vi "Q14070-B030主界面   曲线分布保存.vi"() -> ()   [LabVIEW 2013]
uses:
  <vilib>/printing/EasyPrintingControls.llb/contents.ctl
  <vilib>/printing/EasyPrintingControls.llb/report_type.ctl
  <vilib>/Utility/NIReport.llb/NI_report.lvclass
  <vilib>/printing/EasyPrinting.llb/Easy Print VI Panel or Documentation (path).vi
  <vilib>/Utility/file.llb/Write To Spreadsheet File (DBL).vi
  PCI8622_32.dll
  <vilib>/Utility/NIReport.llb/NI_ReportGenerationCore.lvlib
panel:
  in  "返工次数":dbl
  in  "结束时间":string
  in  "开始时间":string
  out "本工位合格":bool
  out "本工位完成":bool
  out "压衬套伺服压装速度":dbl
  out "压衬套伺服快进速度":dbl
  out "压垫片伺服压装速度":dbl
  out "压垫片伺服快进速度":dbl
  out "压轴承伺服压装速度":dbl
  out "压轴承伺服快进速度":dbl
  in  "本工位放行 7":bool
  in  "本工位放行 6":bool
  in  "本工位放行 5":bool
  in  "本工位放行 4":bool
  in  "压轴承快进位至压装位":bool
  in  "压轴承原位至快进位":bool
  out "压衬套手动走位设置":dbl
  out "压垫片手动走位设置":dbl
  out "压轴承手动走位设置":dbl
  in  "轴承上料工步":u32 caption="工步号1"
  out "轴承上料工步提示":string
  out "压衬套伺服压装位置":dbl
  out "压衬套伺服快进位置":dbl
  out "压垫片伺服压装位置":dbl
  out "压垫片伺服快进位置":dbl
  out "压轴承伺服压装位置":dbl
  out "压轴承伺服快进位置":dbl
  out "压轴承伺服压头位置":dbl
  out "error out":errorcluster
  out "压衬套参数保存错误":errorcluster
  out "压垫片参数保存错误":errorcluster
  in  "压轴承停止完成":bool
  in  "压垫片停止完成":bool
  in  "压衬套停止完成":bool
  in  "预压紧气缸复位":bool
  in  "夹爪全体气缸复位":bool
  in  "电动缸全复位":bool
  in  "电动缸全回零":bool
  in  "工位单循环":bool
  out "压衬套压力数组":dbl[](array[numeric])
  out "压衬套位移数组":dbl[](array[numeric])
  out "压垫片压力数组":dbl[](array[numeric])
  out "压垫片位移数组":dbl[](array[numeric])
  out "压轴承位移数组":dbl[](array[numeric])
  out "压轴承压力数组":dbl[](array[numeric])
  out "压衬套位移":dbl format="%#.3g"
  out "压衬套压力":dbl format="%#.3g"
  out "压垫片位移":dbl format="%#.3g"
  out "压垫片压力":dbl format="%#.3g"
  out "压轴承位移":dbl format="%#.3g"
  out "压轴承压力":dbl format="%#.3g"
  in  "产品ID字符串位数":dbl
  out "报警工步号":u32 caption="工步号1"
  out "报警提示":string
  in  "产品ID":string="201209190001"
  in  "员工ID":string
  out "员工姓名":string
  out "压轴承参数保存错误":errorcluster
  out "传感器保存错误":errorcluster
  in  "报警清除":bool
  in  "参数加载":bool
  in  "型号选择":u32(ring) items=["J706", "J709"]
  out "参数加载错误":errorcluster
  in  "停止":bool
  out "ADODB._Connection Out":refnum<k7>
  out "参数查询错误":errorcluster
  in  "联线按钮":bool
  out "通讯状态":bool
  in  "选项卡控件":T1(tab)
  out "压轴承换向压力(KN)":dbl format="%#.1f"
  out "压轴承压力报警":bool
  out "压轴承监控点压力2(mm)":dbl format="%#.2f"
  out "压轴承监控点压力1(mm)":dbl format="%#.2f"
  out "压轴承区域最大位移1(mm)":dbl format="%#.1f"
  out "压轴承区域最小位移1(mm)":dbl format="%#.1f"
  out "压轴承区域最大压力1(KN)":dbl format="%#.3f"
  out "压轴承区域最小压力1(KN)":dbl format="%#.3f"
  out "压轴承区域最大位移2(mm)":dbl format="%#.1f"
  out "压轴承区域最小位移2(mm)":dbl format="%#.1f"
  out "压轴承区域最大压力2(KN)":dbl format="%#.3f"
  out "压轴承区域最小压力2(KN)":dbl format="%#.3f"
  out "压轴承监控点最小压力1(KN)":dbl format="%#.3f"
  out "压轴承监控点最大压力1(KN)":dbl format="%#.3f"
  out "压轴承监控点最小压力2(KN)":dbl format="%#.3f"
  out "压轴承监控点最大压力2(KN)":dbl format="%#.3f"
  out "压轴承监控点位移1(mm)":dbl format="%#.2f"
  out "压轴承监控点位移2(mm)":dbl format="%#.2f"
  out "压轴承最终压入位移(mm)":dbl format="%#.1f"
  out "压轴承压力曲线":cluster{"Y":dbl[], "Y":dbl[]}[](graph) caption="压球涨堵头1"
  in  "压轴承工步号":u32 caption="工步号1"
  out "压轴承工步提示":string
  out "压轴承压装合格":bool
  out "压轴承压装不合格":bool
  out "压轴承工作完成":bool
  out "压垫片换向压力(KN)":dbl format="%#.1f"
  out "压垫片压力报警":bool
  out "压垫片监控点压力2(mm)":dbl format="%#.2f"
  out "压垫片监控点压力1(mm)":dbl format="%#.2f"
  out "压垫片区域最大位移1(mm)":dbl format="%#.1f"
  out "压垫片区域最小位移1(mm)":dbl format="%#.1f"
  out "压垫片区域最大压力1(KN)":dbl format="%#.3f"
  out "压垫片区域最小压力1(KN)":dbl format="%#.3f"
  out "压垫片区域最大位移2(mm)":dbl format="%#.1f"
  out "压垫片区域最小位移2(mm)":dbl format="%#.1f"
  out "压垫片区域最大压力2(KN)":dbl format="%#.3f"
  out "压垫片区域最小压力2(KN)":dbl format="%#.3f"
  out "压垫片监控点最小压力1(KN)":dbl format="%#.3f"
  out "压垫片监控点最大压力1(KN)":dbl format="%#.3f"
  out "压垫片监控点最小压力2(KN)":dbl format="%#.3f"
  out "压垫片监控点最大压力2(KN)":dbl format="%#.3f"
  out "压垫片监控点位移1(mm)":dbl format="%#.2f"
  out "压垫片监控点位移2(mm)":dbl format="%#.2f"
  out "压垫片最终压入位移(mm)":dbl format="%#.1f"
  out "压垫片压力曲线":cluster{"Y":dbl[], "Y":dbl[]}[](graph) caption="压球涨堵头1"
  in  "压垫片工步号":u32 caption="工步号1"
  out "压垫片工步提示":string
  out "压垫片压装合格":bool
  out "压垫片压装不合格":bool
  out "压垫片工作完成":bool
  out "压衬套换向压力(KN)":dbl format="%#.1f"
  out "压衬套压力报警":bool
  out "压衬套监控点压力2(mm)":dbl format="%#.2f"
  out "压衬套监控点压力1(mm)":dbl format="%#.2f"
  out "压衬套区域最大位移1(mm)":dbl format="%#.1f"
  out "压衬套区域最小位移1(mm)":dbl format="%#.1f"
  out "压衬套区域最大压力1(KN)":dbl format="%#.3f"
  out "压衬套区域最小压力1(KN)":dbl format="%#.3f"
  out "压衬套区域最大位移2(mm)":dbl format="%#.1f"
  out "压衬套区域最小位移2(mm)":dbl format="%#.1f"
  out "压衬套区域最大压力2(KN)":dbl format="%#.3f"
  out "压衬套区域最小压力2(KN)":dbl format="%#.3f"
  out "压衬套监控点最小压力1(KN)":dbl format="%#.3f"
  out "压衬套监控点最大压力1(KN)":dbl format="%#.3f"
  out "压衬套监控点最小压力2(KN)":dbl format="%#.3f"
  out "压衬套监控点最大压力2(KN)":dbl format="%#.3f"
  out "压衬套监控点位移1(mm)":dbl format="%#.2f"
  out "压衬套监控点位移2(mm)":dbl format="%#.2f"
  out "压衬套最终压入位移(mm)":dbl format="%#.1f"
  out "压衬套压力曲线":cluster{"Y":dbl[], "Y":dbl[]}[](graph) caption="压球涨堵头1"
  in  "压衬套工步号":u32 caption="工步号1"
  out "压衬套工步提示":string
  out "压衬套压装合格":bool
  out "压衬套压装不合格":bool
  out "压衬套工作完成":bool
  in  "本工位阻挡":bool
  in  "本工位放行":bool
  in  "本工位阻挡":bool
  in  "上阻挡放行":bool
  in  "流水线顶升原位":bool
  in  "流水线顶升进位":bool
  in  "流水线旋转原位":bool
  in  "流水线旋转进位":bool
  out "上工位放行":bool
  out "本工位放行":bool
  out "旋转盘顶升进位":bool
  out "旋转盘顶升原位":bool
  out "旋转盘旋转进位":bool
  out "旋转盘旋转原位":bool
  out "流水线放行":bool
  out "流水线复位":bool
  out "旋转盘气缸旋转进位检测":bool
  out "流水线急停":bool
  out "旋转盘气缸顶升进位检测":bool
  out "旋转盘气缸顶升原位检测":bool
  out "旋转盘气缸旋转原位检测":bool
  out "本工位检测":bool
  out "下工位检测":bool
  in  "图像识别手动测试":bool
  out "图像识别启动":bool
  out "壳体涂脂阀":bool
  out "压轴涂脂阀":bool
  out "绿灯":bool
  out "黄灯":bool
  out "红灯":bool
  out "衬套在位检测":bool
  out "图像识别反":bool
  out "图像识别正":bool
  out "涂脂按钮":bool
  out "复位":bool
  out "光幕":bool
  out "手/自动":bool
  out "急停":bool
  out "压轴承启动按钮":bool
  out "压垫片启动按钮":bool
  out "压衬套启动按钮":bool
  in  "M夹爪旋转气缸中间位":bool
  out "预压紧气缸2下压":bool
  out "预压紧气缸2上升":bool
  out "预压紧气缸2下位":bool
  out "预压紧气缸2上位":bool
  out "预压紧气缸1下压":bool
  out "预压紧气缸1上升":bool
  out "预压紧气缸1下位":bool
  out "预压紧气缸1上位":bool
  in  "M预压紧气缸2下降":bool
  in  "M预压紧气缸2上升":bool
  in  "M预压紧气缸1下降":bool
  in  "M预压紧气缸1上升":bool
  in  "M夹爪夹紧气缸夹紧":bool
  in  "M夹爪夹紧气缸松开":bool
  in  "M夹爪旋转气缸旋转":bool
  in  "M夹爪旋转气缸回原":bool
  in  "M夹爪翻转气缸翻转":bool
  in  "M夹爪翻转气缸回原":bool
  out "推轴承气缸收回":bool
  out "推轴承气缸推进":bool
  out "推轴承气缸原位":bool
  out "推轴承气缸进位":bool
  in  "M夹爪上升气缸上升":bool
  in  "M夹爪上升气缸下降":bool
  out "夹爪上升气缸上升":bool
  out "夹爪上升气缸下降":bool
  out "夹爪翻转气缸翻转":bool
  out "夹爪夹紧气缸夹紧":bool
  out "夹爪旋转气缸旋转":bool
  out "夹爪旋转气缸回原":bool
  out "夹爪翻转气缸回原":bool
  out "夹爪夹紧气缸松开":bool
  out "夹爪夹紧气缸松开位":bool
  out "夹爪旋转气缸原位":bool
  out "夹爪旋转气缸旋转位":bool
  out "夹爪夹紧气缸夹紧位":bool
  out "夹爪翻转气缸原位":bool
  out "夹爪翻转气缸翻转位":bool
  out "夹爪上升气缸下位":bool
  out "夹爪上升气缸上位":bool
  out "机构气缸当前位置":string[](array[string])
  out "机构气缸当前状态":string[](array[string])
  in  "M推轴承气缸收回":bool
  in  "M推轴承气缸推进":bool
  in  "压衬套手动走位":dbl
  in  "压垫片手动走位":dbl
  in  "压轴承手动走位":dbl
  out "压衬套伺服当前位置":dbl
  out "压垫片伺服当前位置":dbl
  out "压轴承伺服当前位置":dbl
  in  "压衬套手动走位":bool
  in  "压垫片伺服手动走位":bool
  in  "电动缸3下降":bool
  in  "压衬套伺服上升":bool
  in  "电动缸3回零":bool
  in  "电动缸3复位":bool
  in  "压轴承伺服下降":bool
  in  "压轴承伺服上升":bool
  in  "压轴承伺服回零":bool
  in  "压轴承伺服复位":bool
  in  "压垫片伺服下降":bool
  in  "压垫片伺服上升":bool
  in  "压垫片伺服回零":bool
  in  "压垫片伺服复位":bool
  in  "压轴承伺服手动走位":bool
  in  "传感器参数查询":bool
  in  "压衬套压力零点偏移值":dbl format="%#.3f"
  in  "压衬套压力比例偏移值":dbl format="%#.3f"
  in  "压衬套位移比例偏移值":dbl format="%#.3f"
  in  "压衬套位移零点偏移值":dbl format="%#.3f"
  in  "传感器参数保存":bool
  in  "压轴承压力零点偏移值":dbl format="%#.3f"
  in  "压轴承压力比例偏移值":dbl format="%#.3f"
  in  "压轴承位移比例偏移值":dbl format="%#.3f"
  in  "压轴承位移零点偏移值":dbl format="%#.3f"
  in  "压垫片压力零点偏移值":dbl format="%#.3f"
  in  "压垫片压力比例偏移值":dbl format="%#.3f"
  in  "压垫片位移比例偏移值":dbl format="%#.3f"
  in  "压垫片位移零点偏移值":dbl format="%#.3f"
  in  "参数保存":bool
  in  "参数查询":bool
  in  "参数列表":string[][](table)
  # "Q140730-B030 壳体总成装配上线"
  # "Copying (C) 2015 湖北唯思凌科装备制造有限公司 版权所有"
  # "伺服调整位置供调测确定坐标用，正常生产时 禁止操作！！！"
  # "传感器校验区"
  # "关于传感器校验：\n1、传感器校验需要由具备资质的单位或部门进行校验。\n2、具备权限的用户才能够修改传感器校验参数和试验参数。\n3、修改校验参数方法：先将比例偏移置为1，修改零点偏移，使零点值与校验的传感器一致；然后根据增幅调整比例偏移。"
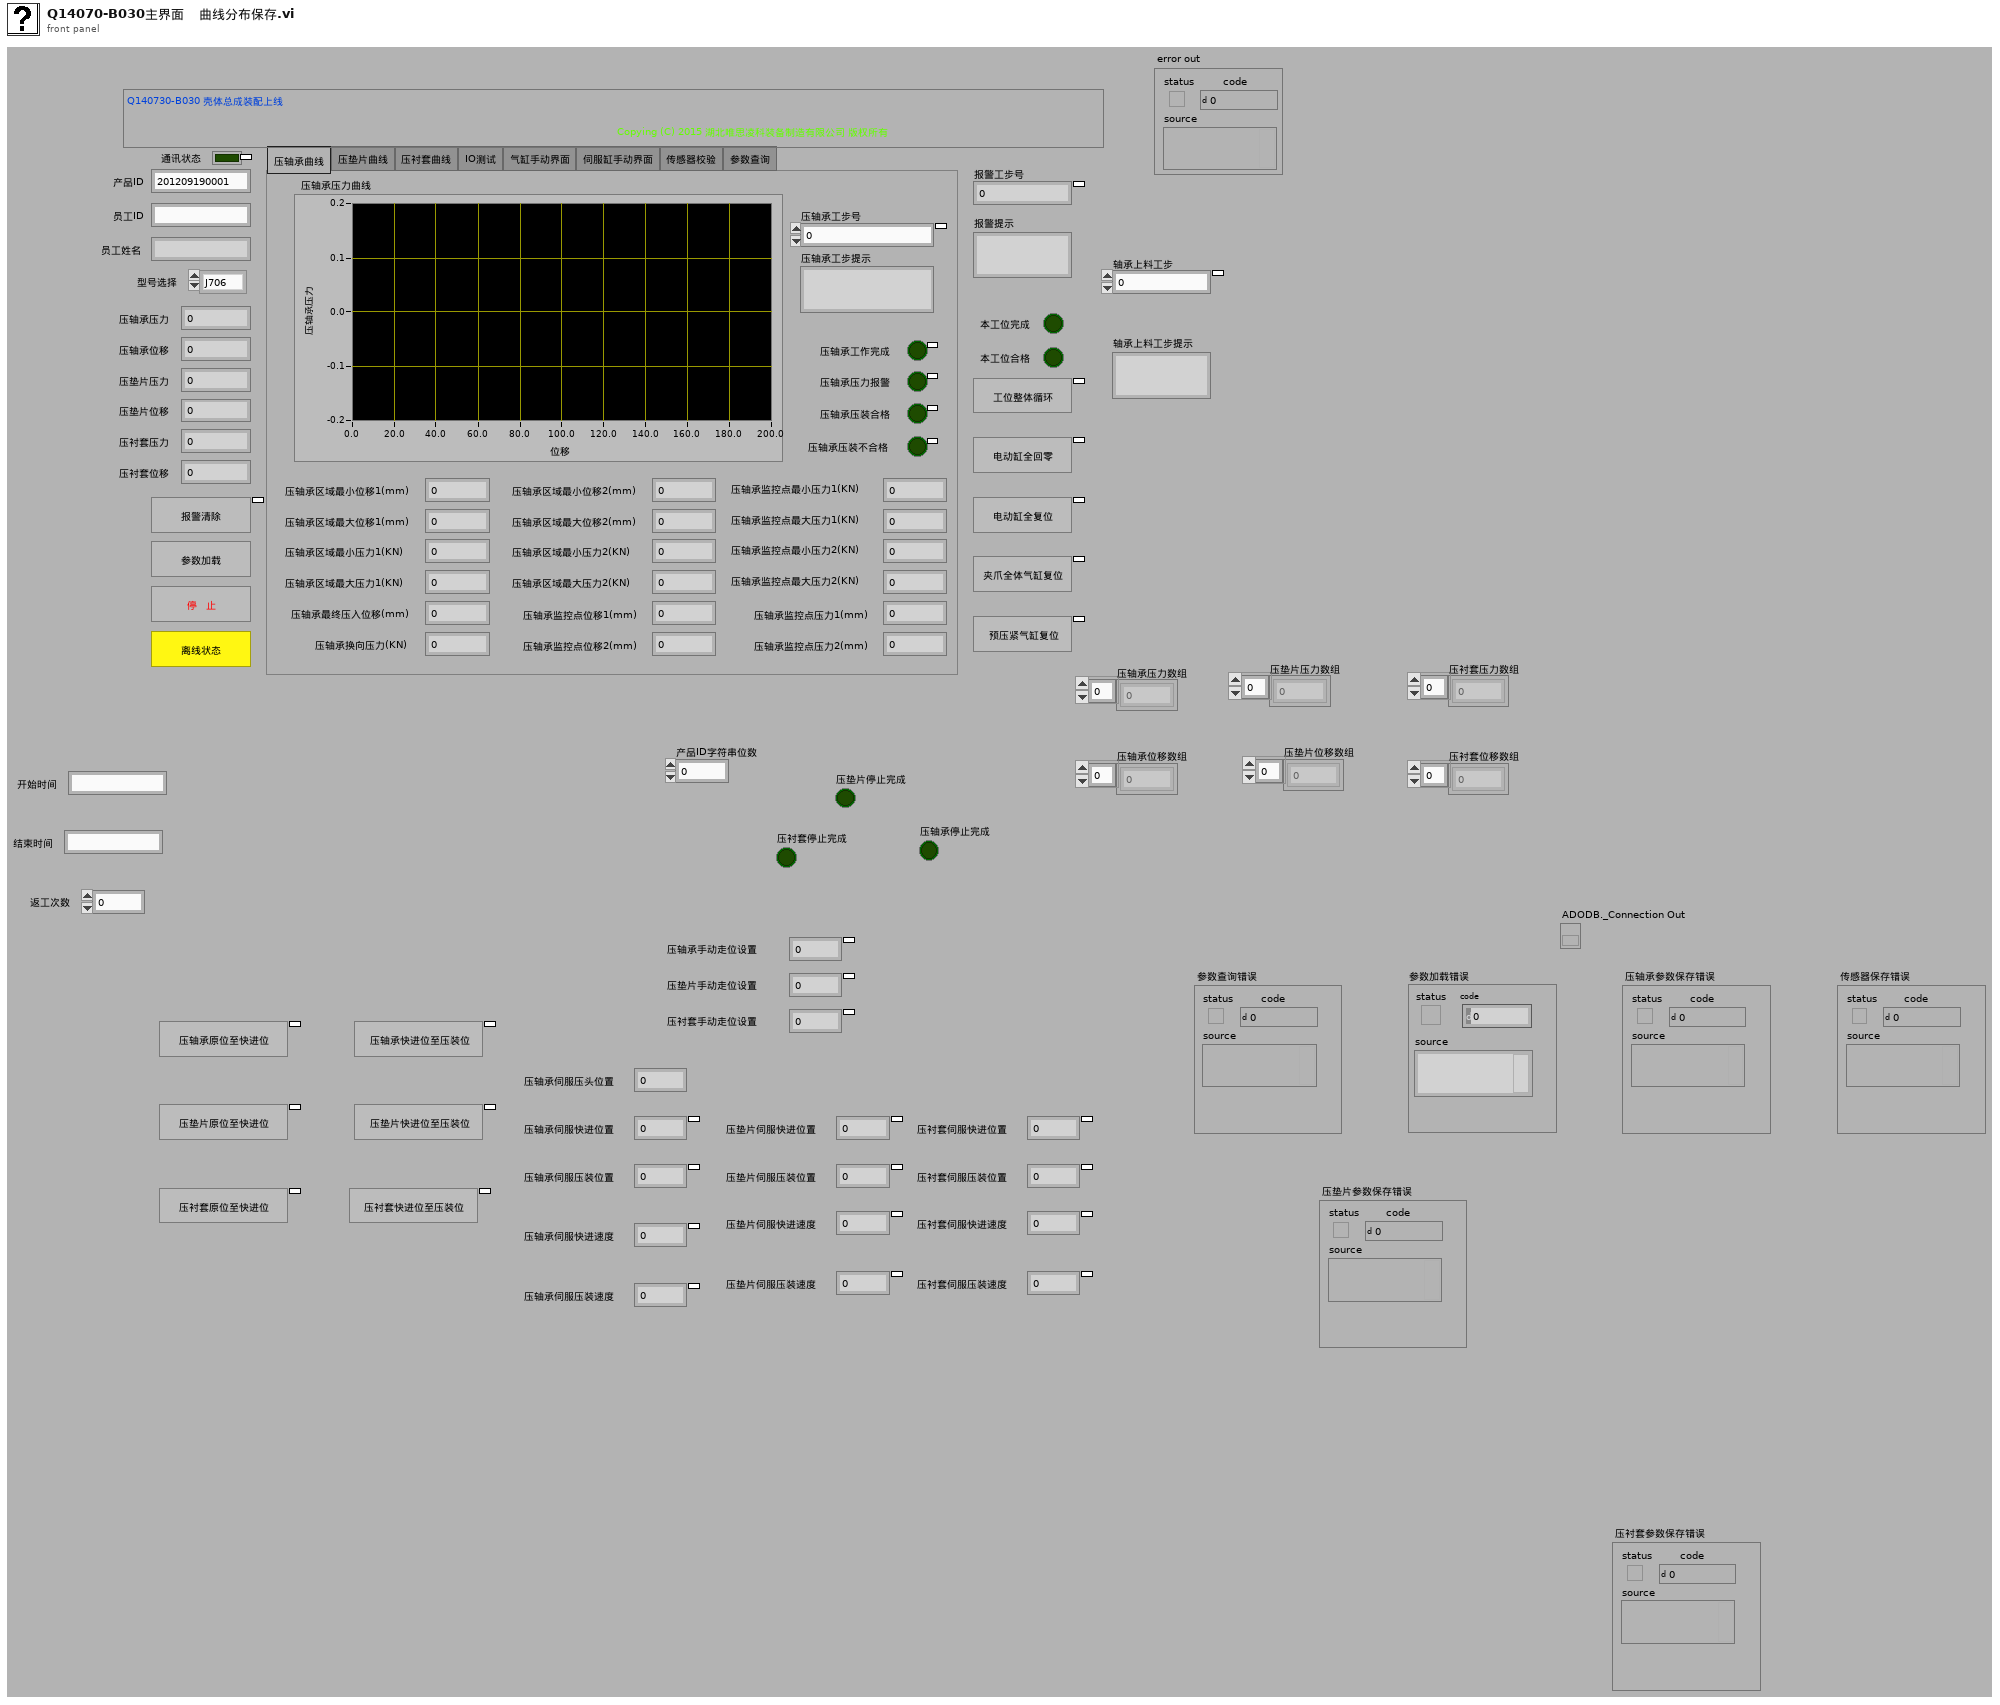
[diagram p1: front panel]
types:
  T1 = enum32{"压轴承曲线", "压垫片曲线", "压衬套曲线", "IO测试", "气缸手动界面", "伺服缸手动界面", "传感器校验", "参数查询"}
  T2 = enum32{"invalid app kind", "Development System", "Run Time System", "Student Edition", "Embedded LabVIEW", "Evaluation", "Custom"}
  T3 = typedef "NI_ReportGenerationCore.lvlib/report_type.ctl" = u16
  T4 = typedef "NI_ReportGenerationCore.lvlib/contents.ctl" = u16
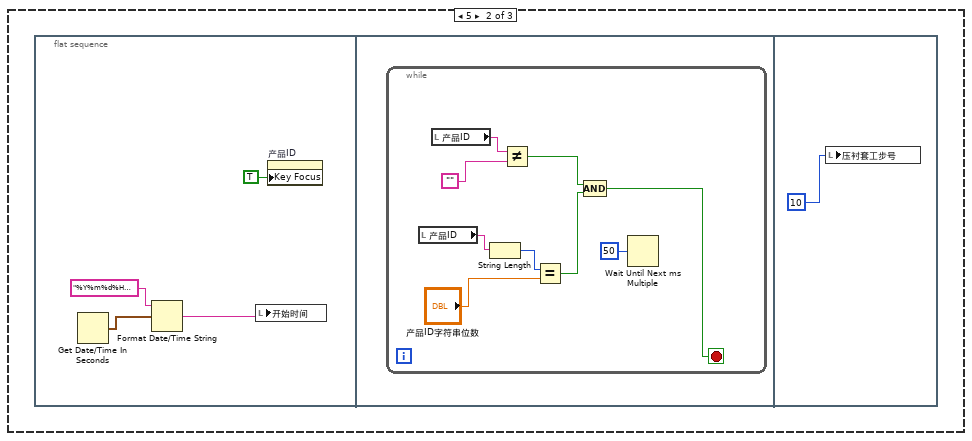
[diagram p3: hidden frame]
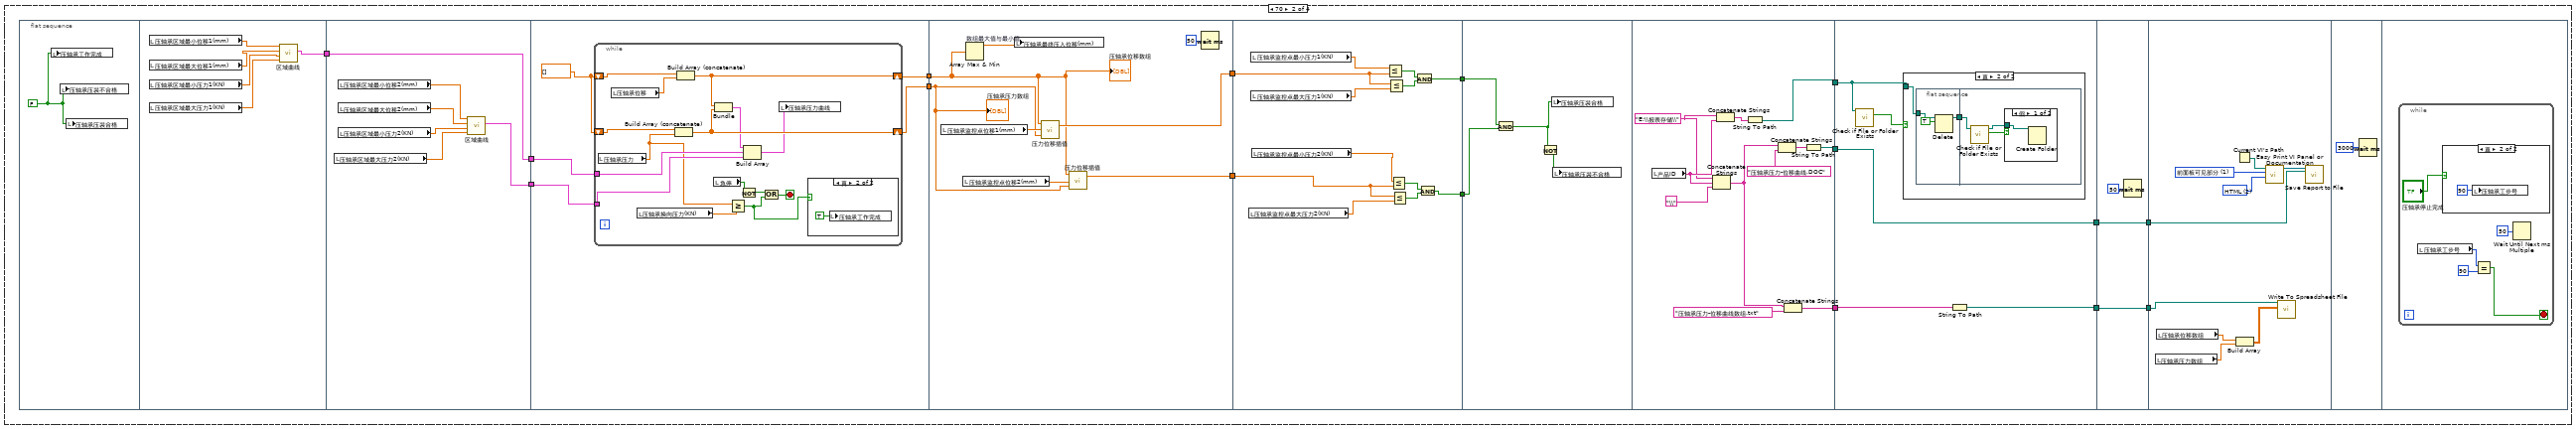
[diagram p10: hidden frame]
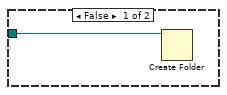
[diagram p12: hidden frame]
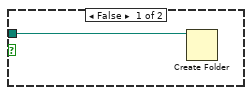
[diagram p15: hidden frame]
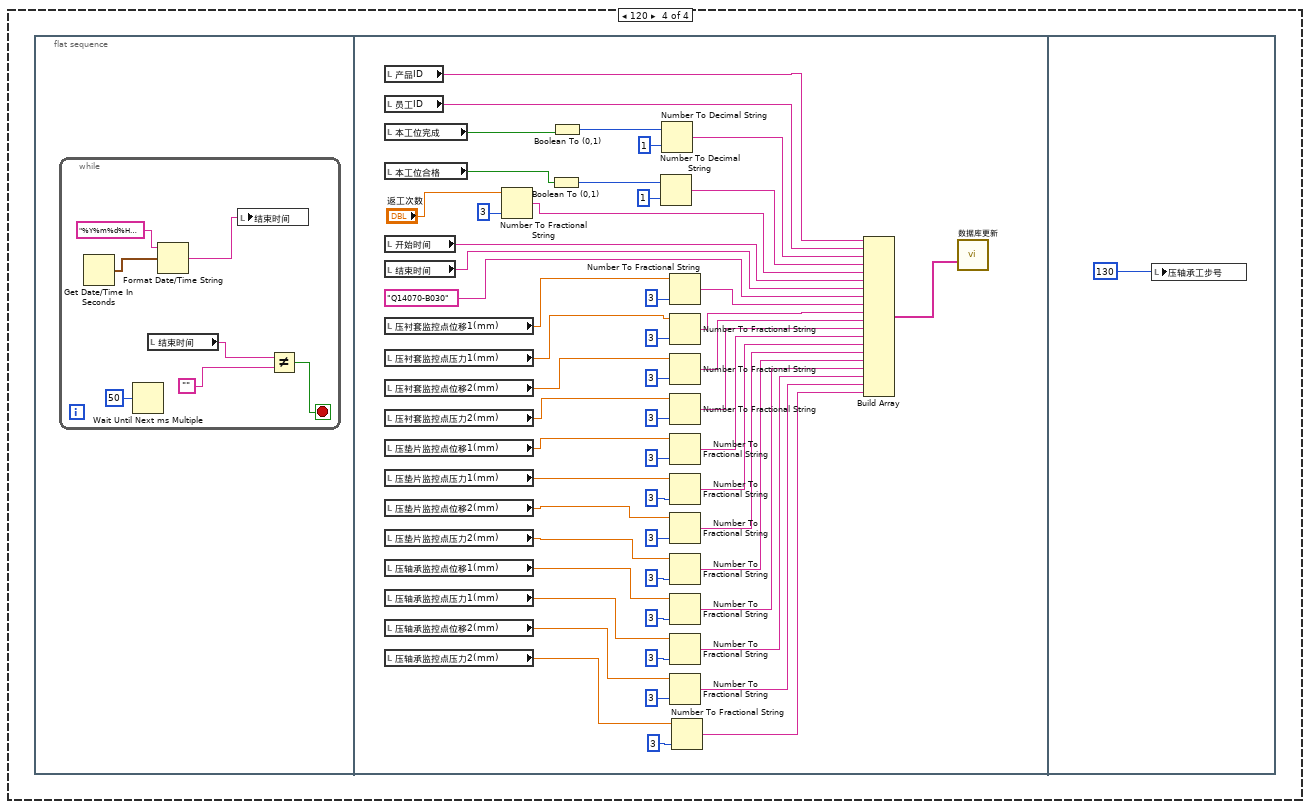
[diagram p17: hidden frame]
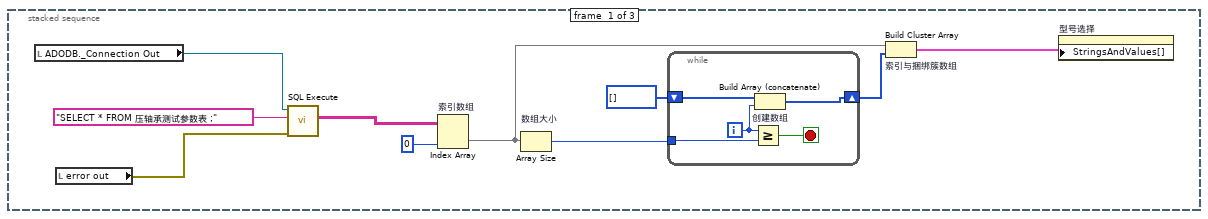
[diagram p19: hidden frame]
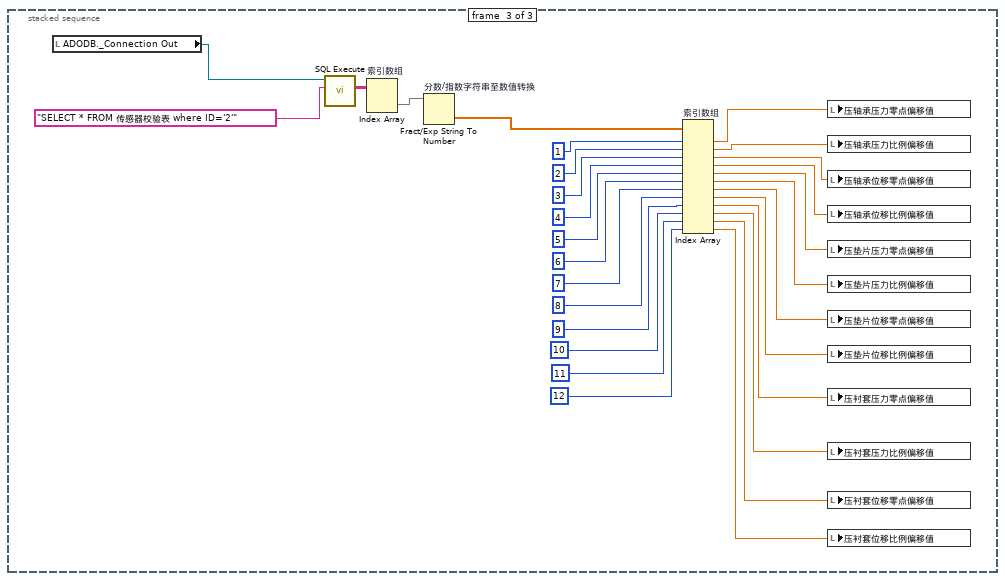
[diagram p20: hidden frame]
diagram:
  n1 = while {
    stop <- w5 stop-if-true
    n2 = event shown="[2] \"参数保存\": 值改变" {
      selector: _ -> [_ _ _ _ _ _]
      dyn-events: _ -> [_ _ _ _ _ _]
      timeout: 500 -> [_ _ _ _ _ _]
      tunnel: [_ _ _ _ _ w268] -> w5
      event Timeout {
        n3 = event-data() -> ()  [unwired: 1 in, 3 out]
      }
      event "参数查询": Value Change {
        n4 = event-data() -> ()  [unwired: 1 in, 6 out]
        n5 = flat-sequence {
          tunnel: [w32] -> w8
          tunnel: [w13] -> w7
          tunnel: w8 -> [w35]
          tunnel: w7 -> [w34]
          frame #0 {
            n6 = call "字符串转换为数组.vi"("查询内容"=",压轴承,压垫片,压衬套") -> ("列首"=w10:string[])  [unwired: 10 in]
            n7 = call "字符串转换为数组.vi"("查询内容"=",产品型号,区域最小位移1,区域最大位移1,区域最小压力1,区域最大压力1,监控点最小压力1,监控点最大压力1,位移监控点1,区域最小位移2,区域最大位移2,区域最小压力2,区域最大压力2,监控点最小压力2,监控点最大压力2,位移监控点2,换向压力,伺服压头位置,伺服快进位置,伺服压装位置,伺服快进速度,伺服压装速度") -> ("列首"=w11:string[])  [unwired: 10 in]
            n8 = property on="参数列表" class="Tbl (严格)"("Row Headers[]"=w11) -> ()  [unwired: 2 in, 2 out]
            n9 = property on="参数列表" class="Tbl (严格)"("Column Headers[]"=w10) -> ()  [unwired: 2 in, 2 out]
          }
          frame #1 {
            n10 = property on="型号选择" class="Ring (严格)"() -> ("RingText.Text"=w26:string)  [unwired: 2 in, 2 out]
            n11 = property on="型号选择" class="Ring (严格)"() -> ("RingText.Text"=w30:string)  [unwired: 2 in, 2 out]
            n12 = property on="型号选择" class="Ring (严格)"() -> ("RingText.Text"=w29:string)  [unwired: 2 in, 2 out]
            n13 = local read "ADODB._Connection Out"() -> (w24:refnum<k7>)
            n14 = local read "ADODB._Connection Out"() -> (w33:refnum<k7>)
            n15 = local read "ADODB._Connection Out"() -> (w27:refnum<k7>)
            n16 = call "创建文本10"("产品型号"=w26) -> ("Result"=w25:string)  [unwired: 13 in, 1 out]
            n17 = call "创建文本"("产品型号"=w30) -> ("Result"=w31:string)  [unwired: 13 in, 1 out]
            n18 = call "创建文本9"("产品型号"=w29) -> ("Result"=w28:string)  [unwired: 13 in, 1 out]
            n19 = call "SQL Execute.vi"("Command Text"=w25, "ADODB._Connection In"=w24) -> ("Data"=w15:string[][])  [unwired: 6 in, 3 out]
            n20 = call "SQL Execute.vi"("Command Text"=w31, "ADODB._Connection In"=w33) -> ("error out"=w32:errorcluster, "Data"=w22:string[][])  [unwired: 6 in, 2 out]
            n21 = call "SQL Execute.vi"("Command Text"=w28, "ADODB._Connection In"=w27) -> ("Data"=w18:string[][])  [unwired: 6 in, 3 out]
            n22 = Index Array(array=w15, index (row)=0 ("索引 (行)")) -> (element=w14:string[])  [unwired: 1 in]
            n23 = Index Array(array=w18, index (row)=0 ("索引 (行)")) -> (element=w17:string[])  [unwired: 1 in]
            n24 = Index Array(array=w22, index (row)=0 ("索引 (行)")) -> (element=w20:string[])  [unwired: 1 in]
            n25 = Build Array(w20, w17, w14) -> (w23:string[][])
            n26 = Transpose 2D Array(2D array=w23) -> (transposed array=w13:string[][])
          }
          frame #2 {
            n27 = local write "参数列表"(w34) -> ()
            "参数查询错误" <- w35
          }
        }
      }
      event "参数保存": Value Change {
        n28 = event-data() -> ()  [unwired: 1 in, 6 out]
        n29 = while {
          i -> [w53]
          stop <- w51 stop-if-true
          n30 = local read "参数列表"() -> (w166:string[][])
          n31 = Greater Or Equal?(x=w53, y=1) -> (x >= y?=w51:bool)
          n32 = Index Array "索引数组"(array=w166, index (col) #1=0 ("禁用的索引 (列)"), index (col) #2=1 ("索引 (列)"), index (col) #3=2 ("索引 (列)")) -> (element #1=w169:string[], element #2=w145:string[], element #3=w126:string[])  [unwired: 3 in]
          n33 = Wait Until Next ms Multiple(millisecond multiple=u32 50 ("毫秒倍数")) -> ()  [unwired: 1 out]
          n34 = Index Array(array=w126, index #1=0 ("索引"), index #2=1 ("索引"), index #3=2 ("索引"), index #4=3 ("索引"), index #5=4 ("索引"), index #6=5 ("索引"), index #7=6 ("索引"), index #8=7 ("索引"), index #9=8 ("索引"), index #10=9 ("索引"), index #11=10 ("索引"), index #12=11 ("索引"), index #13=12 ("索引"), index #14=13 ("索引"), index #15=14 ("索引"), index #16=15 ("索引"), index #18=17 ("索引"), index #19=18 ("索引"), index #20=19 ("索引"), index #21=20 ("索引")) -> (element #1=w40:string, element #2=w71:string, element #3=w70:string, element #4=w69:string, element #5=w68:string, element #6=w67:string, element #7=w66:string, element #8=w65:string, element #9=w64:string, element #10=w63:string, element #11=w62:string, element #12=w61:string, element #13=w60:string, element #14=w59:string, element #15=w58:string, element #16=w57:string, element #18=w56:string, element #19=w55:string, element #20=w37:string, element #21=w36:string)  [unwired: 1 in, 1 out]
          n35 = Index Array(array=w169, index #1=0 ("索引"), index #2=1 ("索引"), index #3=2 ("索引"), index #4=3 ("索引"), index #5=4 ("索引"), index #6=5 ("索引"), index #7=6 ("索引"), index #8=7 ("索引"), index #9=8 ("索引"), index #10=9 ("索引"), index #11=10 ("索引"), index #12=11 ("索引"), index #13=12 ("索引"), index #14=13 ("索引"), index #15=14 ("索引"), index #16=15 ("索引"), index #18=17 ("索引"), index #19=18 ("索引"), index #20=19 ("索引"), index #21=20 ("索引")) -> (element #1=w48:string, element #2=w107:string, element #3=w106:string, element #4=w105:string, element #5=w104:string, element #6=w103:string, element #7=w102:string, element #8=w101:string, element #9=w100:string, element #10=w99:string, element #11=w98:string, element #12=w97:string, element #13=w96:string, element #14=w95:string, element #15=w94:string, element #16=w93:string, element #18=w92:string, element #19=w90:string, element #20=w47:string, element #21=w46:string)  [unwired: 1 in, 1 out]
          n36 = Index Array(array=w145, index #1=0 ("索引"), index #2=1 ("索引"), index #3=2 ("索引"), index #4=3 ("索引"), index #5=4 ("索引"), index #6=5 ("索引"), index #7=6 ("索引"), index #8=7 ("索引"), index #9=8 ("索引"), index #10=9 ("索引"), index #11=10 ("索引"), index #12=11 ("索引"), index #13=12 ("索引"), index #14=13 ("索引"), index #15=14 ("索引"), index #16=15 ("索引"), index #18=17 ("索引"), index #19=18 ("索引"), index #20=19 ("索引"), index #21=20 ("索引")) -> (element #1=w45:string, element #2=w89:string, element #3=w88:string, element #4=w87:string, element #5=w86:string, element #6=w85:string, element #7=w84:string, element #8=w83:string, element #9=w82:string, element #10=w81:string, element #11=w80:string, element #12=w79:string, element #13=w78:string, element #14=w77:string, element #15=w76:string, element #16=w75:string, element #18=w74:string, element #19=w72:string, element #20=w42:string, element #21=w41:string)  [unwired: 1 in, 1 out]
          n37 = call "创建文本5"("压垫片区域最小位移1"=w89, "压垫片区域最大位移1"=w88, "压垫片区域最小压力1"=w87, "压垫片区域最大压力1"=w86, "压垫片监控点最小压力1"=w85, "压垫片监控点最大压力1"=w84, "压垫片位移监控点1"=w83, "压垫片区域最小位移2"=w82, "压垫片区域最大位移2"=w81, "压垫片区域最小压力2"=w80, "压垫片区域最大压力2"=w79, "压垫片监控点最小压力2"=w78, "压垫片监控点最大压力2"=w77, "压垫片位移监控点2"=w76, "压垫片换向压力"=w75, "压垫片伺服快进位置"=w74, "压垫片伺服压装位置"=w72, "压垫片伺服快进速度"=w42, "压垫片伺服压装速度"=w41, "产品型号"=w45) -> ("Result"=w109:string)  [unwired: 6 in, 1 out]
          n38 = call "创建文本6"("压衬套区域最小位移1"=w71, "压衬套区域最大位移1"=w70, "压衬套区域最小压力1"=w69, "压衬套区域最大压力1"=w68, "压衬套监控点最小压力1"=w67, "压衬套监控点最大压力1"=w66, "压衬套位移监控点1"=w65, "压衬套区域最小位移2"=w64, "压衬套区域最大位移2"=w63, "压衬套区域最小压力2"=w62, "压衬套区域最大压力2"=w61, "压衬套监控点最小压力2"=w60, "压衬套监控点最大压力2"=w59, "压衬套位移监控点2"=w58, "压衬套换向压力"=w57, "压衬套伺服快进位置"=w56, "压衬套伺服压装位置"=w55, "压衬套伺服快进速度"=w37, "压衬套伺服压装速度"=w36, "产品型号"=w40) -> ("Result"=w108:string)  [unwired: 6 in, 1 out]
          n39 = call "创建文本3"("压轴承区域最小位移1"=w107, "压轴承区域最大位移1"=w106, "压轴承区域最小压力1"=w105, "压轴承区域最大压力1"=w104, "压轴承监控点最小压力1"=w103, "压轴承监控点最大压力1"=w102, "压轴承位移监控点1"=w101, "压轴承区域最小位移2"=w100, "压轴承区域最大位移2"=w99, "压轴承区域最小压力2"=w98, "压轴承区域最大压力2"=w97, "压轴承监控点最小压力2"=w96, "压轴承监控点最大压力2"=w95, "压轴承位移监控点2"=w94, "压轴承换向压力"=w93, "压轴承伺服快进位置"=w92, "压轴承伺服压装位置"=w90, "压轴承伺服快进速度"=w47, "压轴承伺服压装速度"=w46, "产品型号"=w48) -> ("Result"=w167:string)  [unwired: 6 in, 1 out]
          n40 = call "ADO Connection Create.vi"() -> ("error out"=w114:errorcluster, "ADODB._Connection Out"=w115:refnum<k7>)  [unwired: 10 in]
          n41 = call "ADO Connection Create.vi"() -> ("error out"=w188:errorcluster, "ADODB._Connection Out"=w189:refnum<k7>)  [unwired: 10 in]
          n42 = call "ADO Connection Create.vi"() -> ("error out"=w121:errorcluster, "ADODB._Connection Out"=w120:refnum<k7>)  [unwired: 10 in]
          n43 = call "ADO Connection Open.vi"("error in (no error)"=w114, "ConnectionString"="DSN=参数B030;", "ADODB._Connection In"=w115) -> ("error out"=w111:errorcluster, "ADODB._Connection Out"=w112:refnum<k7>)  [unwired: 7 in]
          n44 = call "ADO Connection Open.vi"("error in (no error)"=w188, "ConnectionString"="DSN=参数B030;", "ADODB._Connection In"=w189) -> ("error out"=w185:errorcluster, "ADODB._Connection Out"=w186:refnum<k7>)  [unwired: 7 in]
          n45 = call "ADO Connection Open.vi"("error in (no error)"=w121, "ConnectionString"="DSN=参数B030;", "ADODB._Connection In"=w120) -> ("error out"=w124:errorcluster, "ADODB._Connection Out"=w123:refnum<k7>)  [unwired: 7 in]
          n46 = call "SQL Execute.vi"("error in (no error)"=w111, "Command Text"=w108, "ADODB._Connection In"=w112) -> ("error out"=w116:errorcluster, "ADODB._Connection Out"=w117:refnum<k7>)  [unwired: 5 in, 2 out]
          n47 = call "SQL Execute.vi"("error in (no error)"=w185, "Command Text"=w167, "ADODB._Connection In"=w186) -> ("error out"=w192:errorcluster, "ADODB._Connection Out"=w193:refnum<k7>)  [unwired: 5 in, 2 out]
          n48 = call "SQL Execute.vi"("error in (no error)"=w124, "Command Text"=w109, "ADODB._Connection In"=w123) -> ("error out"=w119:errorcluster, "ADODB._Connection Out"=w118:refnum<k7>)  [unwired: 5 in, 2 out]
          n49 = call "ADO Connection Close.vi"("error in (no error)"=w116, "ADODB._Connection In"=w117) -> ("error out"=→"压衬套参数保存错误":errorcluster)  [unwired: 8 in, 1 out]
          n50 = call "ADO Connection Close.vi"("error in (no error)"=w192, "ADODB._Connection In"=w193) -> ("error out"=→"压轴承参数保存错误":errorcluster)  [unwired: 8 in, 1 out]
          n51 = call "ADO Connection Close.vi"("error in (no error)"=w119, "ADODB._Connection In"=w118) -> ("error out"=→"压垫片参数保存错误":errorcluster)  [unwired: 8 in, 1 out]
        }
      }
      event "传感器参数查询": Value Change {
        n52 = event-data() -> ()  [unwired: 1 in, 6 out]
        n53 = local read "ADODB._Connection Out"() -> (w202:refnum<k7>)
        n54 = call "SQL Execute.vi"("Command Text"="SELECT * FROM 传感器校验表 where ID='2'", "ADODB._Connection In"=w202) -> ("Data"=w201:string[][])  [unwired: 6 in, 3 out]
        n55 = Index Array "索引数组"(array=w201) -> (element=w200:string[])  [unwired: 2 in]
        n56 = Fract/Exp String To Number "分数/指数字符串至数值转换"(string=w200) -> (number=w199:dbl[])  [unwired: 3 in, 1 out]
        n57 = Index Array "索引数组"(array=w199, index #1=1 ("索引"), index #2=2 ("索引"), index #3=3 ("索引"), index #4=4 ("索引"), index #5=5 ("索引"), index #6=6 ("索引"), index #7=7 ("索引"), index #8=8 ("索引"), index #9=9 ("索引"), index #10=10 ("索引"), index #11=11 ("索引"), index #12=12 ("索引")) -> (element #1=w207:dbl, element #2=w208:dbl, element #3=w209:dbl, element #4=w210:dbl, element #5=w211:dbl, element #6=w212:dbl, element #7=w213:dbl, element #8=w214:dbl, element #9=w219:dbl, element #10=w220:dbl, element #11=w221:dbl, element #12=w222:dbl)
        n58 = local write "压轴承压力零点偏移值"(w207) -> ()
        n59 = local write "压轴承压力比例偏移值"(w208) -> ()
        n60 = local write "压轴承位移零点偏移值"(w209) -> ()
        n61 = local write "压轴承位移比例偏移值"(w210) -> ()
        n62 = local write "压垫片压力零点偏移值"(w211) -> ()
        n63 = local write "压垫片压力比例偏移值"(w212) -> ()
        n64 = local write "压垫片位移零点偏移值"(w213) -> ()
        n65 = local write "压垫片位移比例偏移值"(w214) -> ()
        n66 = local write "压衬套压力零点偏移值"(w219) -> ()
        n67 = local write "压衬套压力比例偏移值"(w220) -> ()
        n68 = local write "压衬套位移零点偏移值"(w221) -> ()
        n69 = local write "压衬套位移比例偏移值"(w222) -> ()
      }
      event "传感器参数保存": Value Change {
        n70 = event-data() -> ()  [unwired: 1 in, 6 out]
        n71 = local read "压轴承压力零点偏移值"() -> (w255:dbl)
        n72 = local read "压轴承压力比例偏移值"() -> (w254:dbl)
        n73 = local read "压轴承位移零点偏移值"() -> (w253:dbl)
        n74 = local read "压轴承位移比例偏移值"() -> (w252:dbl)
        n75 = local read "压垫片压力零点偏移值"() -> (w251:dbl)
        n76 = local read "压垫片压力比例偏移值"() -> (w250:dbl)
        n77 = local read "压垫片位移零点偏移值"() -> (w249:dbl)
        n78 = local read "压垫片位移比例偏移值"() -> (w248:dbl)
        n79 = local read "压衬套压力零点偏移值"() -> (w247:dbl)
        n80 = local read "压衬套压力比例偏移值"() -> (w246:dbl)
        n81 = local read "压衬套位移零点偏移值"() -> (w245:dbl)
        n82 = local read "压衬套位移比例偏移值"() -> (w244:dbl)
        n83 = Number To Fractional String(number=w255, precision (6)=i16 3 ("精度(6)")) -> (F-format string=w243:string)  [unwired: 2 in]
        n84 = Number To Fractional String(number=w254, precision (6)=i16 3 ("精度(6)")) -> (F-format string=w242:string)  [unwired: 2 in]
        n85 = Number To Fractional String(number=w253, precision (6)=i16 3 ("精度(6)")) -> (F-format string=w241:string)  [unwired: 2 in]
        n86 = Number To Fractional String(number=w252, precision (6)=i16 3 ("精度(6)")) -> (F-format string=w240:string)  [unwired: 2 in]
        n87 = Number To Fractional String(number=w251, precision (6)=i16 3 ("精度(6)")) -> (F-format string=w239:string)  [unwired: 2 in]
        n88 = Number To Fractional String(number=w250, precision (6)=i16 3 ("精度(6)")) -> (F-format string=w238:string)  [unwired: 2 in]
        n89 = Number To Fractional String(number=w249, precision (6)=i16 3 ("精度(6)")) -> (F-format string=w237:string)  [unwired: 2 in]
        n90 = Number To Fractional String(number=w248, precision (6)=i16 3 ("精度(6)")) -> (F-format string=w236:string)  [unwired: 2 in]
        n91 = Number To Fractional String(number=w247, precision (6)=i16 3 ("精度(6)")) -> (F-format string=w235:string)  [unwired: 2 in]
        n92 = Number To Fractional String(number=w246, precision (6)=i16 3 ("精度(6)")) -> (F-format string=w234:string)  [unwired: 2 in]
        n93 = Number To Fractional String(number=w245, precision (6)=i16 3 ("精度(6)")) -> (F-format string=w233:string)  [unwired: 2 in]
        n94 = Number To Fractional String(number=w244, precision (6)=i16 3 ("精度(6)")) -> (F-format string=w232:string)  [unwired: 2 in]
        n95 = call "创建文本11"("压轴承压力零点偏移值"=w243, "压轴承压力比例偏移值"=w242, "压轴承位移零点偏移值"=w241, "压轴承位移比例偏移值"=w240, "压垫片压力零点偏移值"=w239, "压垫片压力比例偏移值"=w238, "压垫片位移零点偏移值"=w237, "压垫片位移比例偏移值"=w236, "压衬套压力零点偏移值"=w235, "压衬套压力比例偏移值"=w234, "压衬套位移零点偏移值"=w233, "压衬套位移比例偏移值"=w232) -> ("Result"=w223:string)  [unwired: 14 in, 1 out]
        n96 = call "ADO Connection Create.vi"() -> ("error out"=w230:errorcluster, "ADODB._Connection Out"=w227:refnum<k7>)  [unwired: 10 in]
        n97 = call "ADO Connection Open.vi"("error in (no error)"=w230, "ConnectionString"="DSN=参数B030", "ADODB._Connection In"=w227) -> ("error out"=w231:errorcluster, "ADODB._Connection Out"=w228:refnum<k7>)  [unwired: 7 in]
        n98 = call "SQL Execute.vi"("error in (no error)"=w231, "Command Text"=w223, "ADODB._Connection In"=w228) -> ("error out"=w226:errorcluster, "ADODB._Connection Out"=w225:refnum<k7>)  [unwired: 5 in, 2 out]
        n99 = call "ADO Connection Close.vi"("error in (no error)"=w226, "ADODB._Connection In"=w225) -> ("error out"=→"传感器保存错误":errorcluster)  [unwired: 8 in, 1 out]
      }
      event "停止": Value Change {
        n100 = event-data() -> ()  [unwired: 1 in, 6 out]
        n101 = property on="属性节点" class="App"() -> ("App.Kind"=w269:T2)  [unwired: 2 in, 2 out]
        n102 = case shown="\"Development System\"" w269 {
          tunnel: [_ w270 w271] -> w268
          frame "invalid app kind", Default {
          }
          frame "Development System" {
            w270 = TRUE ("停止？(T)")
            n103 = Stop(stop? (T)=w270) -> ()
          }
          frame "Run Time System" {
            w271 = TRUE ("退出？(T)")
            n104 = Quit LabVIEW(quit? (T)=w271) -> ()
          }
        }
      }
    }
    n105 = Wait Until Next ms Multiple(millisecond multiple=u32 50 ("毫秒倍数")) -> ()  [unwired: 1 out]
  }
  n106 = flat-sequence {
    tunnel: [w272] -> w3
    tunnel: w3 -> [w274]
    tunnel: [w273] -> w2
    tunnel: w2 -> [w368]
    tunnel: [w368] -> w1
    tunnel: w1 -> [w370]
    frame #0 {
      n107 = call "PCI8622配置.vi"() -> ("DeviceID"=w272:i32)  [unwired: 11 in]
    }
    frame #1 {
      n108 = while {
        tunnel: w274 -> [w330]
        tunnel: [w330] -> w273
        stop <- w324 stop-if-true
        w366 = 0  # nRetSizeWords
        w367 = 2048  # nReadSizeWords
        # "hDevice"
        n109 = local read "停止"() -> (w324:bool)
        n110 = Wait Until Next ms Multiple(millisecond multiple=u32 50 ("毫秒倍数")) -> ()  [unwired: 1 out]
        n111 = Initialize Array(u16 0, 2048 ("dimension size")) -> (w359:u16[])
        n112 = dll-call lib="PTH18abs DQ14070B030人机界面-B030PCI8622_32.dll" fn="PCI8622_ReadDeviceProAD_Npt" label="ReadDeviceProAD_Npt"("hDevice"=w330, "ADBuffer[]"=w359, "nReadSizeWords"=w367, "nRetSizeWords"=w366) -> ("ADBuffer[]"=w362:u16[])  [unwired: 7 in, 2 out]
        n113 = Divide(x=w362, y=65536.01) -> (x/y=w363:dbl[])
        n114 = Multiply(x=w363, y=20) -> (x*y=w276:dbl[])
        n115 = Subtract(x=w276, y=10) -> (x-y=w277:dbl[])
        n116 = Decimate 1D Array "抽取一维数组"(w277) -> (w355:dbl[], w345:dbl[], w335:dbl[], w334:dbl[], w286:dbl[], w278:dbl[])  [unwired: 2 out]
        n117 = Add Array Elements(numeric array=w335) -> (sum=w332:dbl)
        n118 = Add Array Elements(numeric array=w355) -> (sum=w356:dbl)
        n119 = Array Size(array=w335) -> (size(s)=w344:i32)
        n120 = Add Array Elements(numeric array=w345) -> (sum=w351:dbl)
        n121 = Add Array Elements(numeric array=w278) -> (sum=w297:dbl)
        n122 = Array Size(array=w355) -> (size(s)=w357:i32)
        n123 = Array Size(array=w345) -> (size(s)=w352:i32)
        n124 = Array Size(array=w278) -> (size(s)=w298:i32)
        n125 = Add Array Elements(numeric array=w334) -> (sum=w331:dbl)
        n126 = Array Size(array=w334) -> (size(s)=w333:i32)
        n127 = Add Array Elements(numeric array=w286) -> (sum=w308:dbl)
        n128 = Array Size(array=w286) -> (size(s)=w307:i32)
        n129 = local read "压轴承压力零点偏移值"() -> (w323:dbl)
        n130 = Divide(x=w332, y=w344) -> (x/y=w343:dbl)
        n131 = Divide(x=w356, y=w357) -> (x/y=w354:dbl)
        n132 = Divide(x=w351, y=w352) -> (x/y=w349:dbl)
        n133 = Divide(x=w297, y=w298) -> (x/y=w302:dbl)
        n134 = Divide(x=w331, y=w333) -> (x/y=w339:dbl)
        n135 = Divide(x=w308, y=w307) -> (x/y=w303:dbl)
        n136 = local read "压轴承位移零点偏移值"() -> (w320:dbl)
        n137 = local read "压垫片压力零点偏移值"() -> (w317:dbl)
        n138 = Subtract(x=w343, y=0.326) -> (x-y=w328:dbl)
        n139 = Subtract(x=w354, y=-0.902) -> (x-y=w283:dbl)
        n140 = Subtract(x=w349, y=0.0) -> (x-y=w347:dbl)
        n141 = Subtract(x=w302, y=0.0) -> (x-y=w296:dbl)
        n142 = Subtract(x=w339, y=0.0) -> (x-y=w326:dbl)
        n143 = local read "压衬套位移零点偏移值"() -> (w294:dbl)
        n144 = Subtract(x=w303, y=0.62) -> (x-y=w309:dbl)
        n145 = local read "压垫片位移零点偏移值"() -> (w319:dbl)
        n146 = local read "压衬套压力零点偏移值"() -> (w311:dbl)
        n147 = Multiply(x=w347, y=25.0) -> (x*y=w346:dbl)
        n148 = Multiply(x=w283, y=500.0) -> (x*y=w282:dbl)
        n149 = Subtract(x=w346, y=w320) -> (x-y=w279:dbl)
        n150 = Multiply(x=w296, y=30.0) -> (x*y=w299:dbl)
        n151 = Multiply(x=w326, y=30.0) -> (x*y=w336:dbl)
        n152 = Multiply(x=w328, y=500.0) -> (x*y=w340:dbl)
        n153 = local read "压轴承位移比例偏移值"() -> (w321:dbl)
        n154 = Multiply(x=w309, y=2000.0) -> (x*y=w306:dbl)
        n155 = Subtract(x=w282, y=w323) -> (x-y=w280:dbl)
        n156 = local read "压垫片压力比例偏移值"() -> (w316:dbl)
        n157 = Subtract(x=w299, y=w294) -> (x-y=w295:dbl)
        n158 = Subtract(x=w336, y=w319) -> (x-y=w325:dbl)
        n159 = Subtract(x=w340, y=w317) -> (x-y=w327:dbl)
        n160 = Subtract(x=w306, y=w311) -> (x-y=w310:dbl)
        n161 = local read "压轴承压力比例偏移值"() -> (w322:dbl)
        n162 = local read "压衬套位移比例偏移值"() -> (w293:dbl)
        n163 = local read "压垫片位移比例偏移值"() -> (w318:dbl)
        n164 = local read "压衬套压力比例偏移值"() -> (w312:dbl)
        n165 = Multiply(x=w279, y=w321) -> (x*y=→"压轴承位移":dbl)
        n166 = Multiply(x=w327, y=w316) -> (x*y=w289:dbl)
        "压垫片压力" <- w289
        n167 = Multiply(x=w280, y=w322) -> (x*y=w315:dbl)
        "压轴承压力" <- w315
        n168 = Multiply(x=w295, y=w293) -> (x*y=→"压衬套位移":dbl)
        n169 = Multiply(x=w325, y=w318) -> (x*y=→"压垫片位移":dbl)
        n170 = Multiply(x=w310, y=w312) -> (x*y=w287:dbl)
        "压衬套压力" <- w287
        n171 = Greater Or Equal?(x=w289, y=6000.0) -> (x >= y?=w285:bool)
        n172 = Greater Or Equal?(x=w315, y=6000.0) -> (x >= y?=w314:bool)
        n173 = local write "压轴承压力报警"(w314) -> ()
        n174 = local write "压垫片压力报警"(w285) -> ()
        n175 = Greater Or Equal?(x=w287, y=22000.0) -> (x >= y?=w284:bool)
        n176 = local write "压衬套压力报警"(w284) -> ()
      }
    }
    frame #2 {
      n177 = dll-call lib="PTH18abs DQ14070B030人机界面-B030PCI8622_32.dll" fn="PCI8622_StopDeviceProAD" label="StopDeviceProAD"("hDevice"=w368) -> ("hDevice"=w369:i32)  [unwired: 4 in, 2 out]
      n178 = dll-call lib="PTH18abs DQ14070B030人机界面-B030PCI8622_32.dll" fn="PCI8622_ReleaseDeviceProAD" label="ReleaseDeviceProAD"("hDevice"=w369) -> ()  [unwired: 5 in, 2 out]
    }
    frame #3 {
      n179 = dll-call lib="PTH18abs DQ14070B030人机界面-B030PCI8622_32.dll" fn="PCI8622_ReleaseDevice" label="ReleaseDevice"("hDevice"=w370) -> ()  [unwired: 5 in, 2 out]
    }
  }
  n180 = while {
    stop <- w371 stop-if-true
    n181 = stacked-sequence {
      frame #0 {
        n182 = Multiply(x="压轴承手动走位", y=-1.0) -> (x*y=→"压轴承手动走位设置":dbl)
        n183 = Multiply(x="压垫片手动走位", y=-1.0) -> (x*y=→"压垫片手动走位设置":dbl)
        n184 = Multiply(x="压衬套手动走位", y=-1.0) -> (x*y=→"压衬套手动走位设置":dbl)
      }
      frame #1 {
        "机构气缸当前位置" <- string[] ["夹爪上升气缸上位", "夹爪上升气缸下位", "夹爪翻转气缸翻转位", "夹爪翻转气缸原位", "夹爪旋转气缸旋转位", "夹爪旋转气缸原位", "夹爪夹紧气缸夹紧位", "夹爪夹紧气缸松开位", "推轴承气缸进位", "推轴承气缸原位", "预压紧气缸1上位", "预压紧气缸1下位", "预压紧气缸2上位", "预压紧气缸2下位"] ("机构气缸当前位置")
        "机构气缸当前状态" <- string[] ["夹爪上升气缸上升", "夹爪上升气缸下降", "夹爪翻转气缸翻转", "夹爪翻转气缸回原", "夹爪旋转气缸旋转", "夹爪旋转气缸回原", "夹爪夹紧气缸夹紧", "夹爪夹紧气缸松开", "推轴承气缸推进", "推轴承气缸收回", "预压紧气缸1上升", "预压紧气缸1下压", "预压紧气缸2上升", "预压紧气缸2下压"] ("机构气缸当前位置")
      }
      frame #2 {
        n185 = case shown="0, 默认" "压轴承工步号" {
          tunnel: ["" ""] -> w401
          frame 0, Default {
          }
          frame 1 {
          }
        }
        "压轴承工步提示" <- w401
        n186 = case shown="0, 默认" "轴承上料工步" {
          tunnel: ["" ""] -> w384
          frame 0, Default {
          }
          frame 1 {
          }
        }
        "轴承上料工步提示" <- w384
        n187 = case shown="0, 默认" "压垫片工步号" {
          tunnel: ["" ""] -> w396
          frame 0, Default {
          }
          frame 1 {
          }
        }
        "压垫片工步提示" <- w396
        n188 = case shown="0, 默认" "压衬套工步号" {
          tunnel: ["" ""] -> w394
          frame 0, Default {
          }
          frame 1 {
          }
        }
        "压衬套工步提示" <- w394
        n189 = local read "报警工步号"() -> (w393:u32)
        n190 = local read "压垫片启动按钮"() -> (w399:bool)
        n191 = local read "绿灯"() -> (w388:bool)
        n192 = local read "压轴承启动按钮"() -> (w389:bool)
        n193 = local read "绿灯"() -> (w386:bool)
        n194 = case shown="0, 默认" w393 {
          tunnel: ["" ""] -> w400
          frame 0, Default {
          }
          frame 1 {
          }
        }
        "报警提示" <- w400
        n195 = Compound Arithmetic op=AND(w389, w388) -> (w390:bool)
        n196 = Compound Arithmetic op=AND(w386, w399) -> (w387:bool)
        n197 = case shown="真" w390 {
          frame False {
          }
          frame True {
            n198 = local write "选项卡控件"(T1."压轴承曲线" ("选项卡控件")) -> ()
          }
        }
        n199 = case shown="真" w387 {
          frame False {
          }
          frame True {
            n200 = local write "选项卡控件"(T1."压垫片曲线" ("选项卡控件")) -> ()
          }
        }
        n201 = local read "压衬套启动按钮"() -> (w398:bool)
        n202 = local read "绿灯"() -> (w391:bool)
        n203 = Compound Arithmetic op=AND(w398, w391) -> (w392:bool)
        n204 = case shown="真" w392 {
          frame False {
          }
          frame True {
            n205 = local write "选项卡控件"(T1."压衬套曲线" ("选项卡控件")) -> ()
          }
        }
      }
    }
    n206 = Wait Until Next ms Multiple(millisecond multiple=u32 50 ("毫秒倍数")) -> ()  [unwired: 1 out]
    n207 = local read "停止"() -> (w371:bool)
  }
  n208 = while {
    stop <- w417 stop-if-true
    n209 = local read "停止"() -> (w417:bool)
    n210 = local read "压衬套工步号"() -> (w418:u32)
    n211 = Wait Until Next ms Multiple(millisecond multiple=u32 50 ("毫秒倍数")) -> ()  [unwired: 1 out]
    n212 = case shown="50" w418 {
      frame 0, Default {
      }
      frame 5 {
        n213 = flat-sequence {
          frame #0 {
            n214 = Get Date/Time In Seconds() -> (seconds since 1Jan1904=w421:timestamp)
            n215 = Format Date/Time String(time format string (%c)="%Y%m%d%H%M" ("时间格式字符串(%c)"), seconds (now)=w421) -> (date/time string=w419:string)  [unwired: 1 in]
            n216 = local write "开始时间"(w419) -> ()
            n217 = property on="产品ID" class="Str"("Key Focus"=TRUE ("键选中")) -> ()  [unwired: 2 in, 2 out]
          }
          frame #1 {
            n218 = while {
              stop <- w425 stop-if-true
              n219 = local read "产品ID"() -> (w429:string)
              n220 = local read "产品ID"() -> (w431:string)
              n221 = String Length(string=w429) -> (length=w428:i32)
              n222 = Not Equal?(x=w431, y="") -> (x != y?=w426:bool)
              n223 = Equal?(x=w428, y="产品ID字符串位数") -> (x = y?=w427:bool)
              n224 = Compound Arithmetic op=AND(w426, w427) -> (w425:bool)
              n225 = Wait Until Next ms Multiple(millisecond multiple=u32 50 ("毫秒倍数")) -> ()  [unwired: 1 out]
            }
          }
          frame #2 {
            n226 = local write "压衬套工步号"(u32 10 ("压轴承工步号")) -> ()
          }
        }
      }
      frame 50 {
        n227 = flat-sequence {
          tunnel: [w449] -> w447
          tunnel: w447 -> [w459]
          tunnel: [w459] -> w446
          tunnel: [w458] -> w445
          tunnel: w446 -> [w463]
          tunnel: w445 -> [w462]
          tunnel: [w461] -> w444
          tunnel: [w460] -> w443
          tunnel: w444 -> [w481]
          tunnel: w443 -> [w486]
          tunnel: [w485] -> w442
          tunnel: [w484] -> w441
          tunnel: w442 -> [w493]
          tunnel: w441 -> [w492]
          tunnel: [w490] -> w440
          tunnel: [w489] -> w439
          tunnel: w440 -> [w503]
          tunnel: w439 -> [w504]
          tunnel: [w506] -> w438
          tunnel: [w505] -> w433
          tunnel: w438 -> [w516]
          tunnel: [w516] -> w436
          tunnel: [w514] -> w434
          tunnel: w433 -> [w515]
          tunnel: [w518] -> w437
          tunnel: w436 -> [w518]
          tunnel: [w517] -> w435
          tunnel: w434 -> [w517]
          tunnel: w437 -> [w524]
          tunnel: w435 -> [w523]
          frame #0 {
            w448 = FALSE ("压轴承压装不合格")
            n228 = local write "压衬套工作完成"(w448) -> ()
            n229 = local write "压衬套压装不合格"(w448) -> ()
            n230 = local write "压衬套压装合格"(w448) -> ()
          }
          frame #1 {
            n231 = local read "压衬套区域最小位移1(mm)"() -> (w453:dbl)
            n232 = local read "压衬套区域最大位移1(mm)"() -> (w452:dbl)
            n233 = local read "压衬套区域最小压力1(KN)"() -> (w451:dbl)
            n234 = local read "压衬套区域最大压力1(KN)"() -> (w450:dbl)
            n235 = call "区域曲线.vi"("区域最大压力(N)"=w450, "区域最小压力(N)"=w451, "区域最大位移(mm)"=w452, "区域最小位移(mm)"=w453) -> ("区域曲线"=w449:cluster{dbl[], dbl[]})  [unwired: 7 in]
          }
          frame #2 {
            n236 = local read "压衬套区域最大压力2(KN)"() -> (w454:dbl)
            n237 = local read "压衬套区域最小位移2(mm)"() -> (w457:dbl)
            n238 = local read "压衬套区域最大位移2(mm)"() -> (w456:dbl)
            n239 = local read "压衬套区域最小压力2(KN)"() -> (w455:dbl)
            n240 = call "区域曲线.vi"("区域最大压力(N)"=w454, "区域最小压力(N)"=w455, "区域最大位移(mm)"=w456, "区域最小位移(mm)"=w457) -> ("区域曲线"=w458:cluster{dbl[], dbl[]})  [unwired: 7 in]
          }
          frame #3 {
            w464 = dbl[] [] ("添加的数组")
            n241 = while {
              shift-right: [w476] -> w461
              shift-left: w464 -> [w479]
              shift-right: [w475] -> w460
              shift-left: w464 -> [w477]
              tunnel: w463 -> [w472]
              tunnel: w462 -> [w471]
              stop <- w466 stop-if-true
              n242 = local read "压衬套压力"() -> (w469:dbl)
              n243 = local read "压衬套位移"() -> (w478:dbl)
              n244 = local read "压衬套换向压力(KN)"() -> (w470:dbl)
              n245 = Build Array (concatenate)(w477, w469) -> (w475:dbl[])
              n246 = Build Array (concatenate)(w479, w478) -> (w476:dbl[])
              n247 = local read "急停"() -> (w468:bool)
              n248 = Bundle(w476, w475) -> (w474:cluster{dbl[], dbl[]})  [unwired: 1 in]
              n249 = Greater Or Equal?(x=w469, y=w470) -> (x >= y?=w465:bool)
              n250 = Not(x=w468) -> (.not. x?=w467:bool)
              n251 = Build Array(w474, w472, w471) -> (w473:cluster{dbl[], dbl[]}[])
              n252 = Compound Arithmetic op=OR(w467, w465) -> (w466:bool)
              n253 = local write "压衬套压力曲线"(w473) -> ()
              n254 = case shown="真" w465 {
                frame False {
                }
                frame True {
                  n255 = local write "压衬套工作完成"(TRUE ("压轴承工作完成")) -> ()
                }
              }
            }
          }
          frame #4 {
            n256 = local read "压衬套监控点位移1(mm)"() -> (w488:dbl)
            n257 = local read "压衬套监控点位移2(mm)"() -> (w487:dbl)
            n258 = Array Max & Min "数组最大值与最小值"(array=w481) -> (max value=w483:dbl)  [unwired: 3 out]
            n259 = local write "压衬套最终压入位移(mm)"(w483) -> ()
            n260 = call "压力位移插值.vi"("压力数组"=w486, "监控点位移"=w488, "位移数组"=w481) -> ("监控点压力"=w485:dbl)  [unwired: 2 in]
            n261 = call "压力位移插值.vi"("压力数组"=w486, "监控点位移"=w487, "位移数组"=w481) -> ("监控点压力"=w484:dbl)  [unwired: 2 in]
            n262 = Wait (ms)(milliseconds to wait=u32 50 ("等待时间（毫秒）")) -> ()  [unwired: 1 out]
            "压衬套压力数组" <- w486
            "压衬套位移数组" <- w481
          }
          frame #5 {
            n263 = local read "压衬套监控点最大压力2(KN)"() -> (w491:dbl)
            n264 = local read "压衬套监控点最小压力1(KN)"() -> (w496:dbl)
            n265 = local read "压衬套监控点最大压力1(KN)"() -> (w494:dbl)
            n266 = local read "压衬套监控点最小压力2(KN)"() -> (w495:dbl)
            n267 = Less Or Equal?(x=w496, y=w493) -> (x <= y?=w500:bool)
            n268 = Less Or Equal?(x=w493, y=w494) -> (x <= y?=w499:bool)
            n269 = Less Or Equal?(x=w495, y=w492) -> (x <= y?=w497:bool)
            n270 = Less Or Equal?(x=w492, y=w491) -> (x <= y?=w498:bool)
            n271 = And(x=w500, y=w499) -> (x .and. y?=w490:bool)
            n272 = And(x=w497, y=w498) -> (x .and. y?=w489:bool)
          }
          frame #6 {
            n273 = And(x=w503, y=w504) -> (x .and. y?=w502:bool)
            n274 = Not(x=w502) -> (.not. x?=w501:bool)
            n275 = local write "压衬套压装合格"(w502) -> ()
            n276 = local write "压衬套压装不合格"(w501) -> ()
          }
          frame #7 {
            n277 = local read "产品ID"() -> (w513:string)
            n278 = Concatenate Strings("E:\\报表存储\\" ("字符串"), w513, "\\" ("字符串")) -> (w511:string)
            n279 = Concatenate Strings(w511, "压衬套压力-位移曲线.DOC" ("字符串")) -> (w507:string)
            n280 = Concatenate Strings(w511, "压衬套压力-位移曲线数组.txt" ("字符串")) -> (w505:string)
            n281 = String To Path(string=w507) -> (path=w506:path)
          }
          frame #8 {
            n282 = String To Path(string=w515) -> (path=w514:path)
          }
          frame #9 {
            n283 = Wait (ms)(milliseconds to wait=u32 50 ("等待时间（毫秒）")) -> ()  [unwired: 1 out]
          }
          frame #10 {
            w527 = T3 2 items=["快速打印", "标准报表", "HTML", "双字节", "Excel"] ("report type (Quick Print)")
            w526 = T4 1 items=["完整前面板", "前面板可见部分", "图标、说明、前面板和程序框图", "说明信息: 使用前面板", "说明信息: 作为子VI使用", "说明信息: 完整", "说明信息: 自定义"] ("contents (complete front panel)")
            n284 = local read "压衬套压力数组"() -> (w521:dbl[])
            n285 = local read "压衬套位移数组"() -> (w522:dbl[])
            n286 = Current VI's Path() -> (path=w525:path)
            n287 = Build Array(w522, w521) -> (w520:dbl[][])
            n288 = call-poly <vilib>:"Easy Print VI Panel or Documentation.vi"("report type (Quick Print)"=w527, "contents (complete front panel)"=w526, "VI path"=w525) -> ("report out"=w528:refnum<class "NI_report.lvclass">)  [unwired: 1 in, 7 out]
            n289 = call-poly <vilib>:"Write To Spreadsheet File.vi"("2D data"=w520, "file path (dialog if empty)"=w523) -> ()  [unwired: 6 in, 1 out]
            n290 = call-dynamic "Save Report to File.vi"("report in"=w528, "report file path"=w524) -> ()  [unwired: 3 in, 11 out]
          }
          frame #11 {
            n291 = Wait (ms)(milliseconds to wait=u32 50 ("等待时间（毫秒）")) -> ()  [unwired: 1 out]
          }
          frame #12 {
            n292 = while {
              stop <- w530 stop-if-true
              n293 = local read "压衬套工步号"() -> (w532:u32)
              n294 = case shown="真" "压衬套停止完成" {
                frame False {
                }
                frame True {
                  n295 = local write "压衬套工步号"(u32 70 ("压轴承工步号")) -> ()
                }
              }
              n296 = Equal?(x=w532, y=u32 70) -> (x = y?=w530:bool)
              n297 = Wait Until Next ms Multiple(millisecond multiple=u32 50 ("毫秒倍数")) -> ()  [unwired: 1 out]
            }
          }
        }
      }
    }
  }
  n298 = while {
    stop <- w537 stop-if-true
    n299 = local read "停止"() -> (w537:bool)
    n300 = local read "压轴承工步号"() -> (w538:u32)
    n301 = Wait Until Next ms Multiple(millisecond multiple=u32 50 ("毫秒倍数")) -> ()  [unwired: 1 out]
    n302 = case shown="110" w538 {
      frame 0, Default {
      }
      frame 70 {
        n303 = flat-sequence {
          tunnel: [w556] -> w554
          tunnel: w554 -> [w566]
          tunnel: [w566] -> w553
          tunnel: [w565] -> w552
          tunnel: w553 -> [w570]
          tunnel: w552 -> [w569]
          tunnel: [w568] -> w551
          tunnel: [w567] -> w550
          tunnel: w551 -> [w588]
          tunnel: w550 -> [w593]
          tunnel: [w592] -> w549
          tunnel: [w591] -> w548
          tunnel: w549 -> [w600]
          tunnel: w548 -> [w599]
          tunnel: [w597] -> w547
          tunnel: [w596] -> w546
          tunnel: w547 -> [w610]
          tunnel: w546 -> [w611]
          tunnel: [w614] -> w545
          tunnel: [w613] -> w544
          tunnel: [w612] -> w539
          tunnel: w545 -> [w626]
          tunnel: w544 -> [w625]
          tunnel: [w625] -> w542
          tunnel: [w623] -> w540
          tunnel: w539 -> [w624]
          tunnel: [w639] -> w543
          tunnel: w542 -> [w639]
          tunnel: [w638] -> w541
          tunnel: w540 -> [w638]
          tunnel: w543 -> [w645]
          tunnel: w541 -> [w644]
          frame #0 {
            w555 = FALSE ("压轴承压装不合格")
            n304 = local write "压轴承工作完成"(w555) -> ()
            n305 = local write "压轴承压装不合格"(w555) -> ()
            n306 = local write "压轴承压装合格"(w555) -> ()
          }
          frame #1 {
            n307 = local read "压轴承区域最小位移1(mm)"() -> (w560:dbl)
            n308 = local read "压轴承区域最大位移1(mm)"() -> (w559:dbl)
            n309 = local read "压轴承区域最小压力1(KN)"() -> (w558:dbl)
            n310 = local read "压轴承区域最大压力1(KN)"() -> (w557:dbl)
            n311 = call "区域曲线.vi"("区域最大压力(N)"=w557, "区域最小压力(N)"=w558, "区域最大位移(mm)"=w559, "区域最小位移(mm)"=w560) -> ("区域曲线"=w556:cluster{dbl[], dbl[]})  [unwired: 7 in]
          }
          frame #2 {
            n312 = local read "压轴承区域最大压力2(KN)"() -> (w561:dbl)
            n313 = local read "压轴承区域最小位移2(mm)"() -> (w564:dbl)
            n314 = local read "压轴承区域最大位移2(mm)"() -> (w563:dbl)
            n315 = local read "压轴承区域最小压力2(KN)"() -> (w562:dbl)
            n316 = call "区域曲线.vi"("区域最大压力(N)"=w561, "区域最小压力(N)"=w562, "区域最大位移(mm)"=w563, "区域最小位移(mm)"=w564) -> ("区域曲线"=w565:cluster{dbl[], dbl[]})  [unwired: 7 in]
          }
          frame #3 {
            w571 = dbl[] [] ("添加的数组")
            n317 = while {
              shift-right: [w583] -> w568
              shift-left: w571 -> [w586]
              shift-right: [w582] -> w567
              shift-left: w571 -> [w584]
              tunnel: w570 -> [w579]
              tunnel: w569 -> [w578]
              stop <- w573 stop-if-true
              n318 = local read "压轴承压力"() -> (w576:dbl)
              n319 = local read "压轴承位移"() -> (w585:dbl)
              n320 = local read "压轴承换向压力(KN)"() -> (w577:dbl)
              n321 = Build Array (concatenate)(w584, w576) -> (w582:dbl[])
              n322 = Build Array (concatenate)(w586, w585) -> (w583:dbl[])
              n323 = local read "急停"() -> (w575:bool)
              n324 = Bundle(w583, w582) -> (w581:cluster{dbl[], dbl[]})  [unwired: 1 in]
              n325 = Greater Or Equal?(x=w576, y=w577) -> (x >= y?=w572:bool)
              n326 = Not(x=w575) -> (.not. x?=w574:bool)
              n327 = Build Array(w581, w579, w578) -> (w580:cluster{dbl[], dbl[]}[])
              n328 = Compound Arithmetic op=OR(w574, w572) -> (w573:bool)
              n329 = local write "压轴承压力曲线"(w580) -> ()
              n330 = case shown="真" w572 {
                frame False {
                }
                frame True {
                  n331 = local write "压轴承工作完成"(TRUE ("压轴承工作完成")) -> ()
                }
              }
            }
          }
          frame #4 {
            n332 = local read "压轴承监控点位移1(mm)"() -> (w595:dbl)
            n333 = local read "压轴承监控点位移2(mm)"() -> (w594:dbl)
            n334 = Array Max & Min "数组最大值与最小值"(array=w588) -> (max value=w590:dbl)  [unwired: 3 out]
            n335 = local write "压轴承最终压入位移(mm)"(w590) -> ()
            n336 = call "压力位移插值.vi"("压力数组"=w593, "监控点位移"=w595, "位移数组"=w588) -> ("监控点压力"=w592:dbl)  [unwired: 2 in]
            n337 = call "压力位移插值.vi"("压力数组"=w593, "监控点位移"=w594, "位移数组"=w588) -> ("监控点压力"=w591:dbl)  [unwired: 2 in]
            n338 = Wait (ms)(milliseconds to wait=u32 50 ("等待时间（毫秒）")) -> ()  [unwired: 1 out]
            "压轴承压力数组" <- w593
            "压轴承位移数组" <- w588
          }
          frame #5 {
            n339 = local read "压轴承监控点最大压力2(KN)"() -> (w598:dbl)
            n340 = local read "压轴承监控点最小压力1(KN)"() -> (w603:dbl)
            n341 = local read "压轴承监控点最大压力1(KN)"() -> (w601:dbl)
            n342 = local read "压轴承监控点最小压力2(KN)"() -> (w602:dbl)
            n343 = Less Or Equal?(x=w603, y=w600) -> (x <= y?=w607:bool)
            n344 = Less Or Equal?(x=w600, y=w601) -> (x <= y?=w606:bool)
            n345 = Less Or Equal?(x=w602, y=w599) -> (x <= y?=w604:bool)
            n346 = Less Or Equal?(x=w599, y=w598) -> (x <= y?=w605:bool)
            n347 = And(x=w607, y=w606) -> (x .and. y?=w597:bool)
            n348 = And(x=w604, y=w605) -> (x .and. y?=w596:bool)
          }
          frame #6 {
            n349 = And(x=w610, y=w611) -> (x .and. y?=w609:bool)
            n350 = Not(x=w609) -> (.not. x?=w608:bool)
            n351 = local write "压轴承压装合格"(w609) -> ()
            n352 = local write "压轴承压装不合格"(w608) -> ()
          }
          frame #7 {
            w621 = "E:\\报表存储\\" ("字符串")
            n353 = local read "产品ID"() -> (w622:string)
            n354 = Concatenate Strings(w621, w622, "\\" ("字符串")) -> (w620:string)
            n355 = Concatenate Strings(w621, w622) -> (w615:string)
            n356 = String To Path(string=w615) -> (path=w614:path)
            n357 = Concatenate Strings(w620, "压轴承压力-位移曲线.DOC" ("字符串")) -> (w616:string)
            n358 = Concatenate Strings(w620, "压轴承压力-位移曲线数组.txt" ("字符串")) -> (w612:string)
            n359 = String To Path(string=w616) -> (path=w613:path)
          }
          frame #8 {
            n360 = call <vilib>:"Check if File or Folder Exists.vi"("path"=w626) -> ("file or folder exists?"=w627:bool)  [unwired: 8 in, 2 out]
            n361 = case shown="真" w627 {
              tunnel: w626 -> [w628 w629]
              frame False {
                n362 = Create Folder(path (use dialog)=w628) -> ()  [unwired: 2 in, 3 out]
              }
              frame True {
                n363 = flat-sequence {
                  tunnel: w629 -> [w633]
                  tunnel: [w631] -> w630
                  tunnel: w630 -> [w636]
                  frame #0 {
                    n364 = Delete(path (use dialog)=w633, entire hierarchy (F)=TRUE ("整个层次结构(F)")) -> (deleted path=w631:path)  [unwired: 3 in, 2 out]
                  }
                  frame #1 {
                    n365 = call <vilib>:"Check if File or Folder Exists.vi"("path"=w636) -> ("file or folder exists?"=w635:bool, "dup path"=w634:path)  [unwired: 8 in, 1 out]
                    n366 = case shown="假" w635 {
                      tunnel: w634 -> [w637 _]
                      frame False {
                        n367 = Create Folder(path (use dialog)=w637) -> ()  [unwired: 2 in, 3 out]
                      }
                      frame True {
                      }
                    }
                  }
                }
              }
            }
            n368 = String To Path(string=w624) -> (path=w623:path)
          }
          frame #9 {
            n369 = Wait (ms)(milliseconds to wait=u32 50 ("等待时间（毫秒）")) -> ()  [unwired: 1 out]
          }
          frame #10 {
            w648 = T3 2 items=["快速打印", "标准报表", "HTML", "双字节", "Excel"] ("report type (Quick Print)")
            w647 = T4 1 items=["完整前面板", "前面板可见部分", "图标、说明、前面板和程序框图", "说明信息: 使用前面板", "说明信息: 作为子VI使用", "说明信息: 完整", "说明信息: 自定义"] ("contents (complete front panel)")
            n370 = local read "压轴承压力数组"() -> (w642:dbl[])
            n371 = local read "压轴承位移数组"() -> (w643:dbl[])
            n372 = Current VI's Path() -> (path=w646:path)
            n373 = Build Array(w643, w642) -> (w641:dbl[][])
            n374 = call-poly <vilib>:"Easy Print VI Panel or Documentation.vi"("report type (Quick Print)"=w648, "contents (complete front panel)"=w647, "VI path"=w646) -> ("report out"=w649:refnum<class "NI_report.lvclass">)  [unwired: 1 in, 7 out]
            n375 = call-poly <vilib>:"Write To Spreadsheet File.vi"("2D data"=w641, "file path (dialog if empty)"=w644) -> ()  [unwired: 6 in, 1 out]
            n376 = call-dynamic "Save Report to File.vi"("report in"=w649, "report file path"=w645) -> ()  [unwired: 3 in, 11 out]
          }
          frame #11 {
            n377 = Wait (ms)(milliseconds to wait=u32 3000 ("等待时间（毫秒）")) -> ()  [unwired: 1 out]
          }
          frame #12 {
            n378 = while {
              stop <- w651 stop-if-true
              n379 = local read "压轴承工步号"() -> (w653:u32)
              n380 = case shown="真" "压轴承停止完成" {
                frame False {
                }
                frame True {
                  n381 = local write "压轴承工步号"(u32 90 ("压轴承工步号")) -> ()
                }
              }
              n382 = Equal?(x=w653, y=u32 90) -> (x = y?=w651:bool)
              n383 = Wait Until Next ms Multiple(millisecond multiple=u32 50 ("毫秒倍数")) -> ()  [unwired: 1 out]
            }
          }
        }
      }
      frame 110 {
        n384 = flat-sequence {
          tunnel: [w676] -> w675
          tunnel: [w679] -> w674
          tunnel: ["F:\\报表存储\\" ("字符串")] -> w673
          tunnel: w675 -> [w697]
          tunnel: w674 -> [w691]
          tunnel: w673 -> [w696]
          tunnel: [w695] -> w672
          tunnel: [w693] -> w671
          tunnel: [w689] -> w670
          tunnel: [w685] -> w669
          tunnel: [w681] -> w668
          tunnel: w672 -> [w703]
          tunnel: [w704] -> w667
          tunnel: w671 -> [w704]
          tunnel: w670 -> [w702]
          tunnel: [w701] -> w666
          tunnel: [w700] -> w665
          tunnel: w669 -> [w700]
          tunnel: w668 -> [w699]
          tunnel: [w699] -> w664
          tunnel: [w719] -> w663
          tunnel: w667 -> [w719]
          tunnel: w666 -> [w718]
          tunnel: [w718] -> w662
          tunnel: [w717] -> w661
          tunnel: w665 -> [w717]
          tunnel: w664 -> [w716]
          tunnel: [w716] -> w660
          tunnel: w663 -> [w730]
          tunnel: w662 -> [w729]
          tunnel: w661 -> [w726]
          tunnel: [w724] -> w659
          tunnel: w660 -> [w723]
          tunnel: [w721] -> w658
          tunnel: w659 -> [w752]
          tunnel: w658 -> [w751]
          tunnel: [w751] -> w657
          tunnel: w657 -> [w760]
          frame #0 {
            n385 = Get Date/Time In Seconds() -> (seconds since 1Jan1904=w678:timestamp)
            n386 = local read "产品ID"() -> (w679:string)
            n387 = Format Date/Time String(time format string (%c)="%Y%m" ("时间格式字符串(%c)"), seconds (now)=w678) -> (date/time string=w676:string)  [unwired: 1 in]
          }
          frame #1 {
            w692 = "\\" ("字符串")
            n388 = Concatenate Strings(w696, w697, w692, w691, w692, w691) -> (w683:string)
            n389 = Concatenate Strings(w696, w697, w692, w691, w692) -> (w698:string)
            n390 = String To Path(string=w698) -> (path=w695:path)
            n391 = Concatenate Strings(w683, "压轴承曲线.DOC" ("字符串")) -> (w694:string)
            n392 = Concatenate Strings(w683, "压衬套曲线.DOC" ("字符串")) -> (w684:string)
            n393 = Concatenate Strings(w683, "压垫片曲线.DOC" ("字符串")) -> (w687:string)
            n394 = Concatenate Strings(w683, "参数曲线数组.txt" ("字符串")) -> (w689:string)
            n395 = String To Path(string=w694) -> (path=w693:path)
            n396 = String To Path(string=w684) -> (path=w681:path)
            n397 = String To Path(string=w687) -> (path=w685:path)
          }
          frame #2 {
            n398 = call <vilib>:"Check if File or Folder Exists.vi"("path"=w703) -> ("file or folder exists?"=w705:bool)  [unwired: 8 in, 2 out]
            n399 = case shown="真" w705 {
              tunnel: w703 -> [w706 w707]
              frame False {
                n400 = Create Folder(path (use dialog)=w706) -> ()  [unwired: 2 in, 3 out]
              }
              frame True {
                n401 = flat-sequence {
                  tunnel: w707 -> [w711]
                  tunnel: [w709] -> w708
                  tunnel: w708 -> [w714]
                  frame #0 {
                    n402 = Delete(path (use dialog)=w711, entire hierarchy (F)=TRUE ("整个层次结构(F)")) -> (deleted path=w709:path)  [unwired: 3 in, 2 out]
                  }
                  frame #1 {
                    n403 = call <vilib>:"Check if File or Folder Exists.vi"("path"=w714) -> ("file or folder exists?"=w713:bool, "dup path"=w712:path)  [unwired: 8 in, 1 out]
                    n404 = case shown="假" w713 {
                      tunnel: w712 -> [w715 _]
                      frame False {
                        n405 = Create Folder(path (use dialog)=w715) -> ()  [unwired: 2 in, 3 out]
                      }
                      frame True {
                      }
                    }
                  }
                }
              }
            }
            n406 = String To Path(string=w702) -> (path=w701:path)
          }
          frame #3 {
            n407 = Wait (ms)(milliseconds to wait=u32 500 ("毫秒倍数")) -> ()  [unwired: 1 out]
          }
          frame #4 {
            n408 = flat-sequence {
              tunnel: w729 -> [w734]
              tunnel: w730 -> [w735]
              tunnel: [w735] -> w728
              tunnel: [w734] -> w727
              tunnel: w726 -> [w733]
              tunnel: [w733] -> w725
              tunnel: w723 -> [w732]
              tunnel: [w732] -> w722
              tunnel: w728 -> [w745]
              tunnel: w727 -> [w742]
              tunnel: w725 -> [w744]
              tunnel: [w744] -> w724
              tunnel: w722 -> [w743]
              tunnel: [w743] -> w721
              frame #0 {
                n409 = local write "选项卡控件"(T1."压轴承曲线" ("选项卡控件")) -> ()
              }
              frame #1 {
                w748 = T3 2 items=["快速打印", "标准报表", "HTML", "双字节", "Excel"] ("report type (Quick Print)")
                w747 = T4 1 items=["完整前面板", "前面板可见部分", "图标、说明、前面板和程序框图", "说明信息: 使用前面板", "说明信息: 作为子VI使用", "说明信息: 完整", "说明信息: 自定义"] ("contents (complete front panel)")
                n410 = local read "压轴承位移数组"() -> (w741:dbl[])
                n411 = local read "压轴承压力数组"() -> (w740:dbl[])
                n412 = local read "压衬套位移数组"() -> (w739:dbl[])
                n413 = local read "压衬套压力数组"() -> (w738:dbl[])
                n414 = local read "压垫片位移数组"() -> (w737:dbl[])
                n415 = local read "压垫片压力数组"() -> (w736:dbl[])
                n416 = Current VI's Path() -> (path=w746:path)
                n417 = call-poly <vilib>:"Easy Print VI Panel or Documentation.vi"("report type (Quick Print)"=w748, "contents (complete front panel)"=w747, "VI path"=w746) -> ("error out"=w750:errorcluster, "report out"=w749:refnum<class "NI_report.lvclass">)  [unwired: 1 in, 6 out]
                n418 = call-dynamic "Save Report to File.vi"("report in"=w749, "report file path"=w745, "error in (no error)"=w750) -> ()  [unwired: 2 in, 11 out]
                n419 = call "导出曲线数组.vi"("压轴承位移参数"=w741, "压轴承压力参数"=w740, "压衬套位移参数"=w739, "压垫片位移参数"=w738, "压垫片压力参数"=w737, "压衬套力参数"=w736, "file path (dialog if empty)"=w742) -> ()  [unwired: 13 in]
              }
            }
          }
          frame #5 {
            n420 = flat-sequence {
              tunnel: w752 -> [w754]
              frame #0 {
                n421 = local write "选项卡控件"(T1."压垫片曲线" ("选项卡控件")) -> ()
              }
              frame #1 {
                w757 = T3 2 items=["快速打印", "标准报表", "HTML", "双字节", "Excel"] ("report type (Quick Print)")
                w758 = T4 1 items=["完整前面板", "前面板可见部分", "图标、说明、前面板和程序框图", "说明信息: 使用前面板", "说明信息: 作为子VI使用", "说明信息: 完整", "说明信息: 自定义"] ("contents (complete front panel)")
                n422 = Current VI's Path() -> (path=w759:path)
                n423 = call-poly <vilib>:"Easy Print VI Panel or Documentation.vi"("report type (Quick Print)"=w757, "contents (complete front panel)"=w758, "VI path"=w759) -> ("error out"=w755:errorcluster, "report out"=w756:refnum<class "NI_report.lvclass">)  [unwired: 1 in, 6 out]
                n424 = call-dynamic "Save Report to File.vi"("report in"=w756, "report file path"=w754, "error in (no error)"=w755) -> ()  [unwired: 2 in, 11 out]
              }
            }
          }
          frame #6 {
            n425 = flat-sequence {
              tunnel: w760 -> [w762]
              frame #0 {
                n426 = local write "选项卡控件"(T1."压衬套曲线" ("选项卡控件")) -> ()
              }
              frame #1 {
                w765 = T3 2 items=["快速打印", "标准报表", "HTML", "双字节", "Excel"] ("report type (Quick Print)")
                w766 = T4 1 items=["完整前面板", "前面板可见部分", "图标、说明、前面板和程序框图", "说明信息: 使用前面板", "说明信息: 作为子VI使用", "说明信息: 完整", "说明信息: 自定义"] ("contents (complete front panel)")
                n427 = Current VI's Path() -> (path=w767:path)
                n428 = call-poly <vilib>:"Easy Print VI Panel or Documentation.vi"("report type (Quick Print)"=w765, "contents (complete front panel)"=w766, "VI path"=w767) -> ("error out"=w763:errorcluster, "report out"=w764:refnum<class "NI_report.lvclass">)  [unwired: 1 in, 6 out]
                n429 = call-dynamic "Save Report to File.vi"("report in"=w764, "report file path"=w762, "error in (no error)"=w763) -> ()  [unwired: 2 in, 11 out]
              }
            }
          }
          frame #7 {
            n430 = local write "选项卡控件"(T1."压轴承曲线" ("选项卡控件")) -> ()
            n431 = Wait (ms)(milliseconds to wait=u32 50 ("等待时间（毫秒）")) -> ()  [unwired: 1 out]
          }
          frame #8 {
            n432 = local write "压轴承工步号"(u32 120 ("压轴承工步号")) -> ()
          }
        }
      }
      frame 120 {
        n433 = flat-sequence {
          frame #0 {
            n434 = while {
              stop <- w772 stop-if-true
              n435 = Get Date/Time In Seconds() -> (seconds since 1Jan1904=w777:timestamp)
              n436 = Wait Until Next ms Multiple(millisecond multiple=u32 50 ("毫秒倍数")) -> ()  [unwired: 1 out]
              n437 = local read "结束时间"() -> (w773:string)
              n438 = Format Date/Time String(time format string (%c)="%Y%m%d%H%M" ("时间格式字符串(%c)"), seconds (now)=w777) -> (date/time string=w771:string)  [unwired: 1 in]
              n439 = local write "结束时间"(w771) -> ()
              n440 = Not Equal?(x=w773, y="") -> (x != y?=w772:bool)
            }
          }
          frame #1 {
            n441 = local read "产品ID"() -> (w812:string)
            n442 = local read "员工ID"() -> (w811:string)
            n443 = local read "本工位完成"() -> (w826:bool)
            n444 = local read "本工位合格"() -> (w825:bool)
            n445 = local read "开始时间"() -> (w806:string)
            n446 = local read "结束时间"() -> (w805:string)
            n447 = local read "压衬套监控点位移1(mm)"() -> (w803:dbl)
            n448 = local read "压衬套监控点压力1(mm)"() -> (w801:dbl)
            n449 = local read "压衬套监控点位移2(mm)"() -> (w798:dbl)
            n450 = local read "压衬套监控点压力2(mm)"() -> (w796:dbl)
            n451 = local read "压垫片监控点位移1(mm)"() -> (w794:dbl)
            n452 = local read "压垫片监控点压力1(mm)"() -> (w792:dbl)
            n453 = local read "压垫片监控点位移2(mm)"() -> (w790:dbl)
            n454 = local read "压垫片监控点压力2(mm)"() -> (w788:dbl)
            n455 = local read "压轴承监控点位移1(mm)"() -> (w787:dbl)
            n456 = local read "压轴承监控点压力1(mm)"() -> (w783:dbl)
            n457 = local read "压轴承监控点位移2(mm)"() -> (w779:dbl)
            n458 = local read "压轴承监控点压力2(mm)"() -> (w778:dbl)
            n459 = Number To Fractional String(number="返工次数", precision (6)=i16 3 ("精度(6)")) -> (F-format string=w807:string)  [unwired: 2 in]
            n460 = Boolean To (0,1)(Boolean=w825) -> (0, 1=w828:i16)
            n461 = Boolean To (0,1)(Boolean=w826) -> (0, 1=w830:i16)
            n462 = Number To Decimal String(number=w828, width (-)=i16 1 ("宽度(-)")) -> (decimal integer string=w809:string)
            n463 = Number To Decimal String(number=w830, width (-)=i16 1 ("宽度(-)")) -> (decimal integer string=w810:string)
            n464 = Number To Fractional String(number=w803, precision (6)=i16 3 ("精度(6)")) -> (F-format string=w802:string)  [unwired: 2 in]
            n465 = Number To Fractional String(number=w801, precision (6)=i16 3 ("精度(6)")) -> (F-format string=w800:string)  [unwired: 2 in]
            n466 = Number To Fractional String(number=w798, precision (6)=i16 3 ("精度(6)")) -> (F-format string=w799:string)  [unwired: 2 in]
            n467 = Number To Fractional String(number=w796, precision (6)=i16 3 ("精度(6)")) -> (F-format string=w797:string)  [unwired: 2 in]
            n468 = Number To Fractional String(number=w794, precision (6)=i16 3 ("精度(6)")) -> (F-format string=w795:string)  [unwired: 2 in]
            n469 = Number To Fractional String(number=w792, precision (6)=i16 3 ("精度(6)")) -> (F-format string=w793:string)  [unwired: 2 in]
            n470 = Number To Fractional String(number=w790, precision (6)=i16 3 ("精度(6)")) -> (F-format string=w791:string)  [unwired: 2 in]
            n471 = Number To Fractional String(number=w788, precision (6)=i16 3 ("精度(6)")) -> (F-format string=w789:string)  [unwired: 2 in]
            n472 = Number To Fractional String(number=w787, precision (6)=i16 3 ("精度(6)")) -> (F-format string=w786:string)  [unwired: 2 in]
            n473 = Number To Fractional String(number=w783, precision (6)=i16 3 ("精度(6)")) -> (F-format string=w782:string)  [unwired: 2 in]
            n474 = Number To Fractional String(number=w779, precision (6)=i16 3 ("精度(6)")) -> (F-format string=w781:string)  [unwired: 2 in]
            n475 = Number To Fractional String(number=w778, precision (6)=i16 3 ("精度(6)")) -> (F-format string=w780:string)  [unwired: 2 in]
            n476 = Build Array(w812, w811, w810, w809, w807, w806, w805, "Q14070-B030", w802, w800, w799, w797, w795, w793, w791, w789, w786, w782, w781, w780) -> (w814:string[])
            n477 = call "数据库更新.vi"("数据"=w814) -> ()  [unwired: 14 in, 1 out]
          }
          frame #2 {
            n478 = local write "压轴承工步号"(u32 130 ("压轴承工步号")) -> ()
          }
        }
      }
    }
  }
  n479 = while {
    stop <- w833 stop-if-true
    n480 = local read "停止"() -> (w833:bool)
    n481 = local read "压垫片工步号"() -> (w834:u32)
    n482 = Wait Until Next ms Multiple(millisecond multiple=u32 50 ("毫秒倍数")) -> ()  [unwired: 1 out]
    n483 = case shown="40" w834 {
      frame 0, Default {
      }
      frame 40 {
        n484 = flat-sequence {
          tunnel: [w851] -> w849
          tunnel: w849 -> [w861]
          tunnel: [w861] -> w848
          tunnel: [w860] -> w847
          tunnel: w848 -> [w865]
          tunnel: w847 -> [w864]
          tunnel: [w863] -> w846
          tunnel: [w862] -> w845
          tunnel: w846 -> [w883]
          tunnel: w845 -> [w888]
          tunnel: [w887] -> w844
          tunnel: [w886] -> w843
          tunnel: w844 -> [w895]
          tunnel: w843 -> [w894]
          tunnel: [w892] -> w842
          tunnel: [w891] -> w841
          tunnel: w842 -> [w905]
          tunnel: w841 -> [w906]
          tunnel: [w908] -> w840
          tunnel: [w907] -> w835
          tunnel: w840 -> [w918]
          tunnel: [w918] -> w838
          tunnel: [w916] -> w836
          tunnel: w835 -> [w917]
          tunnel: [w920] -> w839
          tunnel: w838 -> [w920]
          tunnel: [w919] -> w837
          tunnel: w836 -> [w919]
          tunnel: w839 -> [w926]
          tunnel: w837 -> [w925]
          frame #0 {
            w850 = FALSE ("压轴承压装不合格")
            n485 = local write "压垫片工作完成"(w850) -> ()
            n486 = local write "压垫片压装不合格"(w850) -> ()
            n487 = local write "压垫片压装合格"(w850) -> ()
          }
          frame #1 {
            n488 = local read "压垫片区域最小位移1(mm)"() -> (w855:dbl)
            n489 = local read "压垫片区域最大位移1(mm)"() -> (w854:dbl)
            n490 = local read "压垫片区域最小压力1(KN)"() -> (w853:dbl)
            n491 = local read "压垫片区域最大压力1(KN)"() -> (w852:dbl)
            n492 = call "区域曲线.vi"("区域最大压力(N)"=w852, "区域最小压力(N)"=w853, "区域最大位移(mm)"=w854, "区域最小位移(mm)"=w855) -> ("区域曲线"=w851:cluster{dbl[], dbl[]})  [unwired: 7 in]
          }
          frame #2 {
            n493 = local read "压垫片区域最大压力2(KN)"() -> (w856:dbl)
            n494 = local read "压垫片区域最小位移2(mm)"() -> (w859:dbl)
            n495 = local read "压垫片区域最大位移2(mm)"() -> (w858:dbl)
            n496 = local read "压垫片区域最小压力2(KN)"() -> (w857:dbl)
            n497 = call "区域曲线.vi"("区域最大压力(N)"=w856, "区域最小压力(N)"=w857, "区域最大位移(mm)"=w858, "区域最小位移(mm)"=w859) -> ("区域曲线"=w860:cluster{dbl[], dbl[]})  [unwired: 7 in]
          }
          frame #3 {
            w866 = dbl[] [] ("添加的数组")
            n498 = while {
              shift-right: [w878] -> w863
              shift-left: w866 -> [w881]
              shift-right: [w877] -> w862
              shift-left: w866 -> [w879]
              tunnel: w865 -> [w874]
              tunnel: w864 -> [w873]
              stop <- w868 stop-if-true
              n499 = local read "压垫片压力"() -> (w871:dbl)
              n500 = local read "压垫片位移"() -> (w880:dbl)
              n501 = local read "压垫片换向压力(KN)"() -> (w872:dbl)
              n502 = Build Array (concatenate)(w879, w871) -> (w877:dbl[])
              n503 = Build Array (concatenate)(w881, w880) -> (w878:dbl[])
              n504 = local read "急停"() -> (w870:bool)
              n505 = Bundle(w878, w877) -> (w876:cluster{dbl[], dbl[]})  [unwired: 1 in]
              n506 = Greater Or Equal?(x=w871, y=w872) -> (x >= y?=w867:bool)
              n507 = Not(x=w870) -> (.not. x?=w869:bool)
              n508 = Build Array(w876, w874, w873) -> (w875:cluster{dbl[], dbl[]}[])
              n509 = Compound Arithmetic op=OR(w869, w867) -> (w868:bool)
              n510 = local write "压垫片压力曲线"(w875) -> ()
              n511 = case shown="真" w867 {
                frame False {
                }
                frame True {
                  n512 = local write "压垫片工作完成"(TRUE ("压轴承工作完成")) -> ()
                }
              }
            }
          }
          frame #4 {
            n513 = local read "压垫片监控点位移1(mm)"() -> (w890:dbl)
            n514 = local read "压垫片监控点位移2(mm)"() -> (w889:dbl)
            n515 = Array Max & Min "数组最大值与最小值"(array=w883) -> (max value=w885:dbl)  [unwired: 3 out]
            n516 = local write "压垫片最终压入位移(mm)"(w885) -> ()
            n517 = call "压力位移插值.vi"("压力数组"=w888, "监控点位移"=w890, "位移数组"=w883) -> ("监控点压力"=w887:dbl)  [unwired: 2 in]
            n518 = call "压力位移插值.vi"("压力数组"=w888, "监控点位移"=w889, "位移数组"=w883) -> ("监控点压力"=w886:dbl)  [unwired: 2 in]
            n519 = Wait (ms)(milliseconds to wait=u32 50 ("等待时间（毫秒）")) -> ()  [unwired: 1 out]
            "压垫片压力数组" <- w888
            "压垫片位移数组" <- w883
          }
          frame #5 {
            n520 = local read "压垫片监控点最大压力2(KN)"() -> (w893:dbl)
            n521 = local read "压垫片监控点最小压力1(KN)"() -> (w898:dbl)
            n522 = local read "压垫片监控点最大压力1(KN)"() -> (w896:dbl)
            n523 = local read "压垫片监控点最小压力2(KN)"() -> (w897:dbl)
            n524 = Less Or Equal?(x=w898, y=w895) -> (x <= y?=w902:bool)
            n525 = Less Or Equal?(x=w895, y=w896) -> (x <= y?=w901:bool)
            n526 = Less Or Equal?(x=w897, y=w894) -> (x <= y?=w899:bool)
            n527 = Less Or Equal?(x=w894, y=w893) -> (x <= y?=w900:bool)
            n528 = And(x=w902, y=w901) -> (x .and. y?=w892:bool)
            n529 = And(x=w899, y=w900) -> (x .and. y?=w891:bool)
          }
          frame #6 {
            n530 = And(x=w905, y=w906) -> (x .and. y?=w904:bool)
            n531 = Not(x=w904) -> (.not. x?=w903:bool)
            n532 = local write "压垫片压装合格"(w904) -> ()
            n533 = local write "压垫片压装不合格"(w903) -> ()
          }
          frame #7 {
            n534 = local read "产品ID"() -> (w915:string)
            n535 = Concatenate Strings("E:\\报表存储\\" ("字符串"), w915, "\\" ("字符串")) -> (w913:string)
            n536 = Concatenate Strings(w913, "压垫片压力-位移曲线.DOC" ("字符串")) -> (w909:string)
            n537 = Concatenate Strings(w913, "压垫片压力-位移曲线数组.txt" ("字符串")) -> (w907:string)
            n538 = String To Path(string=w909) -> (path=w908:path)
          }
          frame #8 {
            n539 = String To Path(string=w917) -> (path=w916:path)
          }
          frame #9 {
            n540 = Wait (ms)(milliseconds to wait=u32 50 ("等待时间（毫秒）")) -> ()  [unwired: 1 out]
          }
          frame #10 {
            w929 = T3 2 items=["快速打印", "标准报表", "HTML", "双字节", "Excel"] ("report type (Quick Print)")
            w928 = T4 1 items=["完整前面板", "前面板可见部分", "图标、说明、前面板和程序框图", "说明信息: 使用前面板", "说明信息: 作为子VI使用", "说明信息: 完整", "说明信息: 自定义"] ("contents (complete front panel)")
            n541 = local read "压垫片压力数组"() -> (w923:dbl[])
            n542 = local read "压垫片位移数组"() -> (w924:dbl[])
            n543 = Current VI's Path() -> (path=w927:path)
            n544 = Build Array(w924, w923) -> (w922:dbl[][])
            n545 = call-poly <vilib>:"Easy Print VI Panel or Documentation.vi"("report type (Quick Print)"=w929, "contents (complete front panel)"=w928, "VI path"=w927) -> ("report out"=w930:refnum<class "NI_report.lvclass">)  [unwired: 1 in, 7 out]
            n546 = call-poly <vilib>:"Write To Spreadsheet File.vi"("2D data"=w922, "file path (dialog if empty)"=w925) -> ()  [unwired: 6 in, 1 out]
            n547 = call-dynamic "Save Report to File.vi"("report in"=w930, "report file path"=w926) -> ()  [unwired: 3 in, 11 out]
          }
          frame #11 {
            n548 = Wait (ms)(milliseconds to wait=u32 50 ("等待时间（毫秒）")) -> ()  [unwired: 1 out]
          }
          frame #12 {
            n549 = while {
              stop <- w932 stop-if-true
              n550 = local read "压垫片工步号"() -> (w934:u32)
              n551 = case shown="真" "压垫片停止完成" {
                frame False {
                }
                frame True {
                  n552 = local write "压垫片工步号"(u32 60 ("压轴承工步号")) -> ()
                }
              }
              n553 = Equal?(x=w934, y=u32 60) -> (x = y?=w932:bool)
              n554 = Wait Until Next ms Multiple(millisecond multiple=u32 50 ("毫秒倍数")) -> ()  [unwired: 1 out]
            }
          }
        }
      }
    }
  }
  n555 = flat-sequence {
    frame #0 {
      n556 = call "ADO Connection Create.vi"() -> ("error out"=w941:errorcluster, "ADODB._Connection Out"=w942:refnum<k7>)  [unwired: 10 in]
      n557 = call "ADO Connection Open.vi"("error in (no error)"=w941, "ConnectionString"="DSN=参数B030;", "ADODB._Connection In"=w942) -> ("error out"=→"error out":errorcluster, "ADODB._Connection Out"=→"ADODB._Connection Out":refnum<k7>)  [unwired: 7 in]
    }
    frame #1 {
      n558 = while {
        stop <- w944 stop-if-true
        n559 = local read "停止"() -> (w944:bool)
        n560 = Wait Until Next ms Multiple(millisecond multiple=u32 100 ("毫秒倍数")) -> ()  [unwired: 1 out]
        n561 = First Call?() -> (First Call?: T/F=w947:bool)
        n562 = Or(x=w947, y="参数加载") -> (x .or. y?=w946:bool)
        n563 = case shown="真" w946 {
          frame False {
          }
          frame True {
            n564 = stacked-sequence {
              frame #0 {
                n565 = local read "ADODB._Connection Out"() -> (w949:refnum<k7>)
                n566 = local read "error out"() -> (w948:errorcluster)
                n567 = call "SQL Execute.vi"("error in (no error)"=w948, "Command Text"="SELECT * FROM 压轴承测试参数表 ;", "ADODB._Connection In"=w949) -> ("Data"=w952:string[][])  [unwired: 5 in, 3 out]
                n568 = Index Array "索引数组"(array=w952, index (col)=0 ("禁用的索引 (列)")) -> (element=w955:string[])  [unwired: 1 in]
                n569 = Array Size "数组大小"(array=w955) -> (size(s)=w954:i32)
                n570 = while {
                  shift-right: [w960] -> w953
                  shift-left: i32[] [] -> [w961]
                  tunnel: w954 -> [w958]
                  i -> [w959]
                  stop <- w962 stop-if-true
                  n571 = Greater Or Equal?(x=w959, y=w958) -> (x >= y?=w962:bool)
                  n572 = Build Array (concatenate) "创建数组"(w961, w959) -> (w960:i32[])
                }
                n573 = Build Cluster Array "索引与捆绑簇数组"(w955, w953) -> (w950:cluster{"String":string, i32}[])
                n574 = property on="型号选择" class="Ring (严格)"("StringsAndValues[]"=w950) -> ()  [unwired: 2 in, 2 out]
              }
              frame #1 {
                n575 = property on="型号选择" class="Ring (严格)"() -> ("RingText.Text"=w1024:string)  [unwired: 2 in, 2 out]
                n576 = property on="型号选择" class="Ring (严格)"() -> ("RingText.Text"=w1066:string)  [unwired: 2 in, 2 out]
                n577 = property on="型号选择" class="Ring (严格)"() -> ("RingText.Text"=w1076:string)  [unwired: 2 in, 2 out]
                n578 = local read "ADODB._Connection Out"() -> (w1023:refnum<k7>)
                n579 = local read "ADODB._Connection Out"() -> (w1065:refnum<k7>)
                n580 = local read "ADODB._Connection Out"() -> (w1077:refnum<k7>)
                n581 = call "创建文本8"("产品型号"=w1024) -> ("Result"=w989:string)  [unwired: 13 in, 1 out]
                n582 = call "创建文本7"("产品型号"=w1066) -> ("Result"=w1031:string)  [unwired: 13 in, 1 out]
                n583 = call "创建文本4"("产品型号"=w1076) -> ("Result"=w1112:string)  [unwired: 13 in, 1 out]
                n584 = local read "error out"() -> (w1025:errorcluster)
                n585 = local read "error out"() -> (w1067:errorcluster)
                n586 = local read "error out"() -> (w1075:errorcluster)
                n587 = call "SQL Execute.vi"("error in (no error)"=w1025, "Command Text"=w989, "ADODB._Connection In"=w1023) -> ("Data"=w987:string[][])  [unwired: 5 in, 3 out]
                n588 = call "SQL Execute.vi"("error in (no error)"=w1067, "Command Text"=w1031, "ADODB._Connection In"=w1065) -> ("Data"=w1029:string[][])  [unwired: 5 in, 3 out]
                n589 = call "SQL Execute.vi"("error in (no error)"=w1075, "Command Text"=w1112, "ADODB._Connection In"=w1077) -> ("Data"=w1114:string[][])  [unwired: 5 in, 3 out]
                n590 = Index Array "索引数组"(array=w987, index (row)=0 ("索引 (行)")) -> (element=w990:string[])  [unwired: 1 in]
                n591 = Index Array "索引数组"(array=w1029, index (row)=0 ("索引 (行)")) -> (element=w1032:string[])  [unwired: 1 in]
                n592 = Index Array "索引数组"(array=w1114, index (row)=0 ("索引 (行)")) -> (element=w1111:string[])  [unwired: 1 in]
                n593 = Fract/Exp String To Number "分数/指数字符串至数值转换"(string=w990) -> (number=w1008:dbl[])  [unwired: 3 in, 1 out]
                n594 = Fract/Exp String To Number "分数/指数字符串至数值转换"(string=w1032) -> (number=w1050:dbl[])  [unwired: 3 in, 1 out]
                n595 = Fract/Exp String To Number "分数/指数字符串至数值转换"(string=w1111) -> (number=w1092:dbl[])  [unwired: 3 in, 1 out]
                n596 = Index Array(array=w1008, index #1=1 ("索引"), index #2=2 ("索引"), index #3=3 ("索引"), index #4=4 ("索引"), index #5=5 ("索引"), index #6=6 ("索引"), index #7=7 ("索引"), index #8=8 ("索引"), index #9=9 ("索引"), index #10=10 ("索引"), index #11=11 ("索引"), index #12=12 ("索引"), index #13=13 ("索引"), index #14=14 ("索引"), index #15=15 ("索引"), index #17=17 ("索引"), index #18=18 ("索引"), index #19=19 ("索引"), index #20=20 ("索引")) -> (element #1=w1009:dbl, element #2=w1010:dbl, element #3=w1011:dbl, element #4=w1012:dbl, element #5=w1013:dbl, element #6=w1014:dbl, element #7=w1015:dbl, element #8=w1016:dbl, element #9=w1017:dbl, element #10=w1018:dbl, element #11=w1019:dbl, element #12=w1020:dbl, element #13=w1021:dbl, element #14=w1022:dbl, element #15=w1026:dbl, element #17=w1027:dbl, element #18=w1028:dbl, element #19=w964:dbl, element #20=w963:dbl)  [unwired: 1 in, 1 out]
                n597 = Index Array(array=w1050, index #1=1 ("索引"), index #2=2 ("索引"), index #3=3 ("索引"), index #4=4 ("索引"), index #5=5 ("索引"), index #6=6 ("索引"), index #7=7 ("索引"), index #8=8 ("索引"), index #9=9 ("索引"), index #10=10 ("索引"), index #11=11 ("索引"), index #12=12 ("索引"), index #13=13 ("索引"), index #14=14 ("索引"), index #15=15 ("索引"), index #17=17 ("索引"), index #18=18 ("索引"), index #19=19 ("索引"), index #20=20 ("索引")) -> (element #1=w1051:dbl, element #2=w1052:dbl, element #3=w1053:dbl, element #4=w1054:dbl, element #5=w1055:dbl, element #6=w1056:dbl, element #7=w1057:dbl, element #8=w1058:dbl, element #9=w1059:dbl, element #10=w1060:dbl, element #11=w1061:dbl, element #12=w1062:dbl, element #13=w1063:dbl, element #14=w1064:dbl, element #15=w1068:dbl, element #17=w1069:dbl, element #18=w1070:dbl, element #19=w967:dbl, element #20=w968:dbl)  [unwired: 1 in, 1 out]
                n598 = local write "压垫片伺服压装速度"(w968) -> ()
                n599 = local write "压垫片伺服快进速度"(w967) -> ()
                n600 = Index Array(array=w1092, index #1=1 ("索引"), index #2=2 ("索引"), index #3=3 ("索引"), index #4=4 ("索引"), index #5=5 ("索引"), index #6=6 ("索引"), index #7=7 ("索引"), index #8=8 ("索引"), index #9=9 ("索引"), index #10=10 ("索引"), index #11=11 ("索引"), index #12=12 ("索引"), index #13=13 ("索引"), index #14=14 ("索引"), index #15=15 ("索引"), index #16=16 ("索引"), index #17=17 ("索引"), index #18=18 ("索引"), index #19=19 ("索引"), index #20=20 ("索引")) -> (element #1=w1091:dbl, element #2=w1090:dbl, element #3=w1089:dbl, element #4=w1088:dbl, element #5=w1087:dbl, element #6=w1086:dbl, element #7=w1085:dbl, element #8=w1084:dbl, element #9=w1083:dbl, element #10=w1082:dbl, element #11=w1081:dbl, element #12=w1080:dbl, element #13=w1079:dbl, element #14=w1078:dbl, element #15=w1074:dbl, element #16=w1073:dbl, element #17=w1072:dbl, element #18=w1071:dbl, element #19=w971:dbl, element #20=w972:dbl)
                n601 = local write "压轴承伺服快进速度"(w971) -> ()
                n602 = local write "压轴承伺服压装速度"(w972) -> ()
                n603 = Multiply(x=-1.0, y=w1070) -> (x*y=w980:dbl)
                n604 = Multiply(x=w1027, y=-1.0) -> (x*y=w978:dbl)
                n605 = Multiply(x=w1071, y=-1.0) -> (x*y=w984:dbl)
                n606 = Multiply(x=-1.0, y=w1069) -> (x*y=w982:dbl)
                n607 = Multiply(x=-1.0, y=w1072) -> (x*y=w986:dbl)
                n608 = Multiply(x=w1028, y=-1.0) -> (x*y=w976:dbl)
                n609 = local write "压衬套伺服快进速度"(w964) -> ()
                n610 = local write "压衬套伺服压装速度"(w963) -> ()
                n611 = local write "压衬套区域最小位移1(mm)"(w1009) -> ()
                n612 = local write "压衬套区域最大位移1(mm)"(w1010) -> ()
                n613 = local write "压衬套区域最小压力1(KN)"(w1011) -> ()
                n614 = local write "压衬套区域最大压力1(KN)"(w1012) -> ()
                n615 = local write "压衬套监控点最小压力1(KN)"(w1013) -> ()
                n616 = local write "压衬套监控点最大压力1(KN)"(w1014) -> ()
                n617 = local write "压衬套监控点位移1(mm)"(w1015) -> ()
                n618 = local write "压衬套区域最小位移2(mm)"(w1016) -> ()
                n619 = local write "压衬套区域最大位移2(mm)"(w1017) -> ()
                n620 = local write "压衬套区域最小压力2(KN)"(w1018) -> ()
                n621 = local write "压衬套区域最大压力2(KN)"(w1019) -> ()
                n622 = local write "压衬套监控点最小压力2(KN)"(w1020) -> ()
                n623 = local write "压衬套监控点最大压力2(KN)"(w1021) -> ()
                n624 = local write "压衬套监控点位移2(mm)"(w1022) -> ()
                n625 = local write "压衬套换向压力(KN)"(w1026) -> ()
                n626 = local write "压衬套伺服快进位置"(w978) -> ()
                n627 = local write "压衬套伺服压装位置"(w976) -> ()
                n628 = local write "压垫片区域最小位移1(mm)"(w1051) -> ()
                n629 = local write "压垫片区域最大位移1(mm)"(w1052) -> ()
                n630 = local write "压垫片区域最小压力1(KN)"(w1053) -> ()
                n631 = local write "压垫片区域最大压力1(KN)"(w1054) -> ()
                n632 = local write "压垫片监控点最小压力1(KN)"(w1055) -> ()
                n633 = local write "压垫片监控点最大压力1(KN)"(w1056) -> ()
                n634 = local write "压垫片监控点位移1(mm)"(w1057) -> ()
                n635 = local write "压垫片区域最小位移2(mm)"(w1058) -> ()
                n636 = local write "压垫片区域最大位移2(mm)"(w1059) -> ()
                n637 = local write "压垫片区域最小压力2(KN)"(w1060) -> ()
                n638 = local write "压垫片区域最大压力2(KN)"(w1061) -> ()
                n639 = local write "压垫片监控点最小压力2(KN)"(w1062) -> ()
                n640 = local write "压垫片监控点最大压力2(KN)"(w1063) -> ()
                n641 = local write "压垫片监控点位移2(mm)"(w1064) -> ()
                n642 = local write "压垫片换向压力(KN)"(w1068) -> ()
                n643 = local write "压垫片伺服快进位置"(w982) -> ()
                n644 = local write "压垫片伺服压装位置"(w980) -> ()
                n645 = local write "压轴承区域最小位移1(mm)"(w1091) -> ()
                n646 = local write "压轴承区域最大位移1(mm)"(w1090) -> ()
                n647 = local write "压轴承区域最小压力1(KN)"(w1089) -> ()
                n648 = local write "压轴承区域最大压力1(KN)"(w1088) -> ()
                n649 = local write "压轴承监控点最小压力1(KN)"(w1087) -> ()
                n650 = local write "压轴承监控点最大压力1(KN)"(w1086) -> ()
                n651 = local write "压轴承监控点位移1(mm)"(w1085) -> ()
                n652 = local write "压轴承区域最小位移2(mm)"(w1084) -> ()
                n653 = local write "压轴承区域最大位移2(mm)"(w1083) -> ()
                n654 = local write "压轴承区域最小压力2(KN)"(w1082) -> ()
                n655 = local write "压轴承区域最大压力2(KN)"(w1081) -> ()
                n656 = local write "压轴承监控点最小压力2(KN)"(w1080) -> ()
                n657 = local write "压轴承监控点最大压力2(KN)"(w1079) -> ()
                n658 = local write "压轴承监控点位移2(mm)"(w1078) -> ()
                n659 = local write "压轴承换向压力(KN)"(w1074) -> ()
                n660 = local write "压轴承伺服压头位置"(w1073) -> ()
                n661 = local write "压轴承伺服快进位置"(w986) -> ()
                n662 = local write "压轴承伺服压装位置"(w984) -> ()
              }
              frame #2 {
                n663 = local read "ADODB._Connection Out"() -> (w1135:refnum<k7>)
                n664 = call "SQL Execute.vi"("Command Text"="SELECT * FROM 传感器校验表 where ID='2'", "ADODB._Connection In"=w1135) -> ("Data"=w1136:string[][])  [unwired: 6 in, 3 out]
                n665 = Index Array "索引数组"(array=w1136) -> (element=w1137:string[])  [unwired: 2 in]
                n666 = Fract/Exp String To Number "分数/指数字符串至数值转换"(string=w1137) -> (number=w1138:dbl[])  [unwired: 3 in, 1 out]
                n667 = Index Array "索引数组"(array=w1138, index #1=1 ("索引"), index #2=2 ("索引"), index #3=3 ("索引"), index #4=4 ("索引"), index #5=5 ("索引"), index #6=6 ("索引"), index #7=7 ("索引"), index #8=8 ("索引"), index #9=9 ("索引"), index #10=10 ("索引"), index #11=11 ("索引"), index #12=12 ("索引")) -> (element #1=w1130:dbl, element #2=w1129:dbl, element #3=w1128:dbl, element #4=w1127:dbl, element #5=w1126:dbl, element #6=w1125:dbl, element #7=w1124:dbl, element #8=w1123:dbl, element #9=w1118:dbl, element #10=w1117:dbl, element #11=w1116:dbl, element #12=w1115:dbl)
                n668 = local write "压轴承压力零点偏移值"(w1130) -> ()
                n669 = local write "压轴承压力比例偏移值"(w1129) -> ()
                n670 = local write "压轴承位移零点偏移值"(w1128) -> ()
                n671 = local write "压轴承位移比例偏移值"(w1127) -> ()
                n672 = local write "压垫片压力零点偏移值"(w1126) -> ()
                n673 = local write "压垫片压力比例偏移值"(w1125) -> ()
                n674 = local write "压垫片位移零点偏移值"(w1124) -> ()
                n675 = local write "压垫片位移比例偏移值"(w1123) -> ()
                n676 = local write "压衬套压力零点偏移值"(w1118) -> ()
                n677 = local write "压衬套压力比例偏移值"(w1117) -> ()
                n678 = local write "压衬套位移零点偏移值"(w1116) -> ()
                n679 = local write "压衬套位移比例偏移值"(w1115) -> ()
              }
            }
          }
        }
      }
    }
    frame #2 {
      n680 = local read "ADODB._Connection Out"() -> (w1145:refnum<k7>)
      n681 = local read "error out"() -> (w1144:errorcluster)
      n682 = call "ADO Connection Close.vi"("error in (no error)"=w1144, "ADODB._Connection In"=w1145) -> ("error out"=→"参数加载错误":errorcluster)  [unwired: 8 in, 1 out]
    }
  }
